vi "Dielectric vs Temperature - freq (4192A).vi"() -> ()   [LabVIEW 2013]
uses:
  <vilib>/Instr/_visa.llb/VISA Configure Serial Port (Instr).vi
  <vilib>/Utility/file.llb/Write To Spreadsheet File (DBL).vi
  Instance           5 32Saved   K vs Temp - freq (4284A) .vi
  Instance           6 32Saved   K vs Temp - freq (4284A) .vi
  Instance          15 32Saved   K vs Temp - freq (4284A) .vi
  Instance          16 32Saved   K vs Temp - freq (4284A) .vi
  Instance           7 32Saved   K vs Temp - freq (4284A) .vi
  Instance           8 32Saved   K vs Temp - freq (4284A) .vi
  Instance           9 32Saved   K vs Temp - freq (4284A) .vi
  Instance          10 32Saved   K vs Temp - freq (4284A) .vi
  Instance          11 32Saved   K vs Temp - freq (4284A) .vi
  Instance          12 32Saved   K vs Temp - freq (4284A) .vi
  Instance          13 32Saved   K vs Temp - freq (4284A) .vi
  Instance          14 32Saved   K vs Temp - freq (4284A) .vi
  Instance          17 32Saved   K vs Temp - freq (4284A) .vi
  Instance          18 32Saved   K vs Temp - freq (4284A) .vi
  Instance          19 32Saved   K vs Temp - freq (4284A) .vi
  Instance          20 32Saved   K vs Temp - freq (4284A) .vi
  Instance          21 32Saved   K vs Temp - freq (4284A) .vi
  Instance          22 32Saved   K vs Temp - freq (4284A) .vi
  Instance          23 32Saved   K vs Temp - freq (4284A) .vi
  Instance          25 32Saved   K vs Temp - freq (4284A) .vi
  Instance          24 32Saved   K vs Temp - freq (4284A) .vi
  Instance          26 32Saved   K vs Temp - freq (4284A) .vi
panel:
  in  "Freq Value (Hz) (1MHz)":dbl=1000000.0
  out "tand1M":dbl
  out "K1M":dbl
  out "C1M":dbl
  out "Temp1MHz":dbl format="%#_3g"
  in  "Freq Value (Hz) (500kHz)":dbl=500000.0
  out "tand500k":dbl
  out "K500k":dbl
  out "C500k":dbl
  out "Temp500kHz":dbl format="%#_3g"
  in  "Freq Value (Hz) (250kHz)":dbl=250000.0
  out "tand250k":dbl
  out "K250k":dbl
  out "C250k":dbl
  out "Temp250kHz":dbl format="%#_3g"
  in  "Freq Value (Hz) (100kHz)":dbl=100000.0
  out "tand100k":dbl
  out "K100k":dbl
  out "C100k":dbl
  out "Temp100kHz":dbl format="%#_3g"
  in  "Freq Value (Hz) (50kHz)":dbl=50000.0
  out "tand50k":dbl
  out "K50k":dbl
  out "C50k":dbl
  out "Temp50kHz":dbl format="%#_3g"
  in  "Freq Value (Hz) (25kHz)":dbl=25000.0
  out "tand25k":dbl
  out "K25k":dbl
  out "C25k":dbl
  out "Temp25kHz":dbl format="%#_3g"
  in  "Freq Value (Hz) (10kHz)":dbl=10000.0
  out "tand10k":dbl
  out "K10k":dbl
  out "C10k":dbl
  out "Temp10kHz":dbl format="%#_3g"
  in  "Freq Value (Hz) (5kHz)":dbl=5000.0
  out "tand5k":dbl
  out "K5k":dbl
  out "C5k":dbl
  out "Temp5kHz":dbl format="%#_3g"
  in  "Freq Value (Hz) (2.5kHz)":dbl=2500.0
  out "tand2.5k":dbl
  out "K2.5k":dbl
  out "C2.5k":dbl
  out "Temp2.5kHz":dbl format="%#_3g"
  in  "Freq Value (Hz) (1kHz)":dbl=1000.0
  out "tand1k":dbl
  out "K1k":dbl
  out "C1k":dbl
  out "Temp1kHz":dbl format="%#_3g"
  in  "tand500k":dbl[](array[numeric])
  in  "K500k":dbl[](array[numeric])
  in  "Temp500k":dbl[](array[numeric])
  out "Temp500Hz":dbl format="%#_3g"
  out "C500":dbl
  out "?":dbl
  out "tand500":dbl
  in  "Freq Value (Hz) (500Hz)":dbl=500.0
  in  "Freq Value (Hz) (250Hz)":dbl=250.0
  in  "Freq Value (Hz) (100Hz)":dbl=100.0
  in  "Freq Value (Hz) (50Hz)":dbl=50.0
  in  "Freq Value (Hz) (25Hz)":dbl=25.0
  in  "tand100k":dbl[](array[numeric])
  in  "tand10k":dbl[](array[numeric])
  in  "tand1k":dbl[](array[numeric])
  in  "tand100":dbl[](array[numeric])
  in  "K100k":dbl[](array[numeric])
  in  "K10k":dbl[](array[numeric])
  in  "K1k":dbl[](array[numeric])
  in  "K100":dbl[](array[numeric])
  in  "Temp100k":dbl[](array[numeric])
  in  "Temp10k":dbl[](array[numeric])
  in  "Temp1k":dbl[](array[numeric])
  in  "Temp100":dbl[](array[numeric])
  out "Temp250Hz":dbl format="%#_3g"
  out "Temp100Hz":dbl format="%#_3g"
  out "tand25":dbl
  out "Temp50Hz":dbl format="%#_3g"
  in  "Start":bool
  out "Thickness":dbl
  out "Area":dbl
  in  "stop":bool
  out "tand250":dbl
  out "tand100":dbl
  out "tand50":dbl
  out "K250":dbl
  out "K100":dbl
  out "K50":dbl
  out "K25":dbl
  out "C250":dbl
  out "C100":dbl
  out "C50":dbl
  out "C25":dbl
  out "Temp25Hz":dbl format="%#_3g"
  out "Dielectric Loss vs. Temperature":cluster{"Y":dbl[], "Y":dbl[]}[](graph)
  out "Relative Permittivity vs. Temperature":cluster{"Y":dbl[], "Y":dbl[]}[](graph)
  in  "Comment (Sample's Name, compositions, whatever you want,..)":string
  in  "Thickness (mm)":dbl
  in  "Diameter (mm)":dbl
  in  "Path & File Name (*.txt)":path
  # "Temperature (C)"
  # "Frequency (Hz)"
  # "Capacitance (F)"
  # "Relative Permittivity"
  # "Dielectric Loss"
  # "Sample Details"
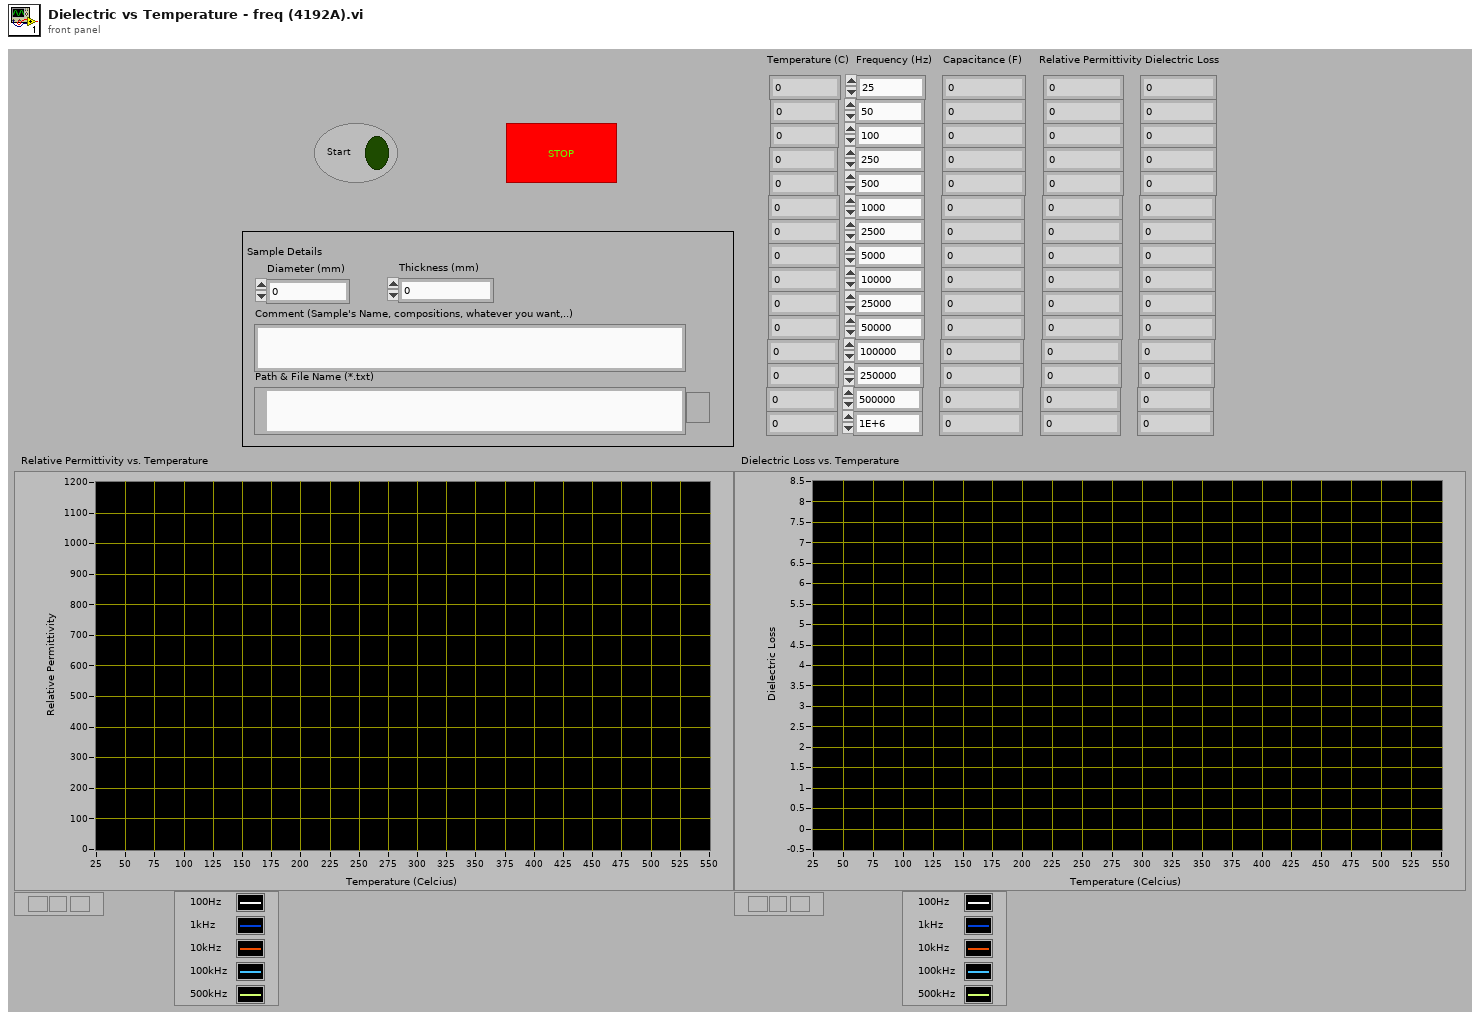
[diagram p1: front panel]
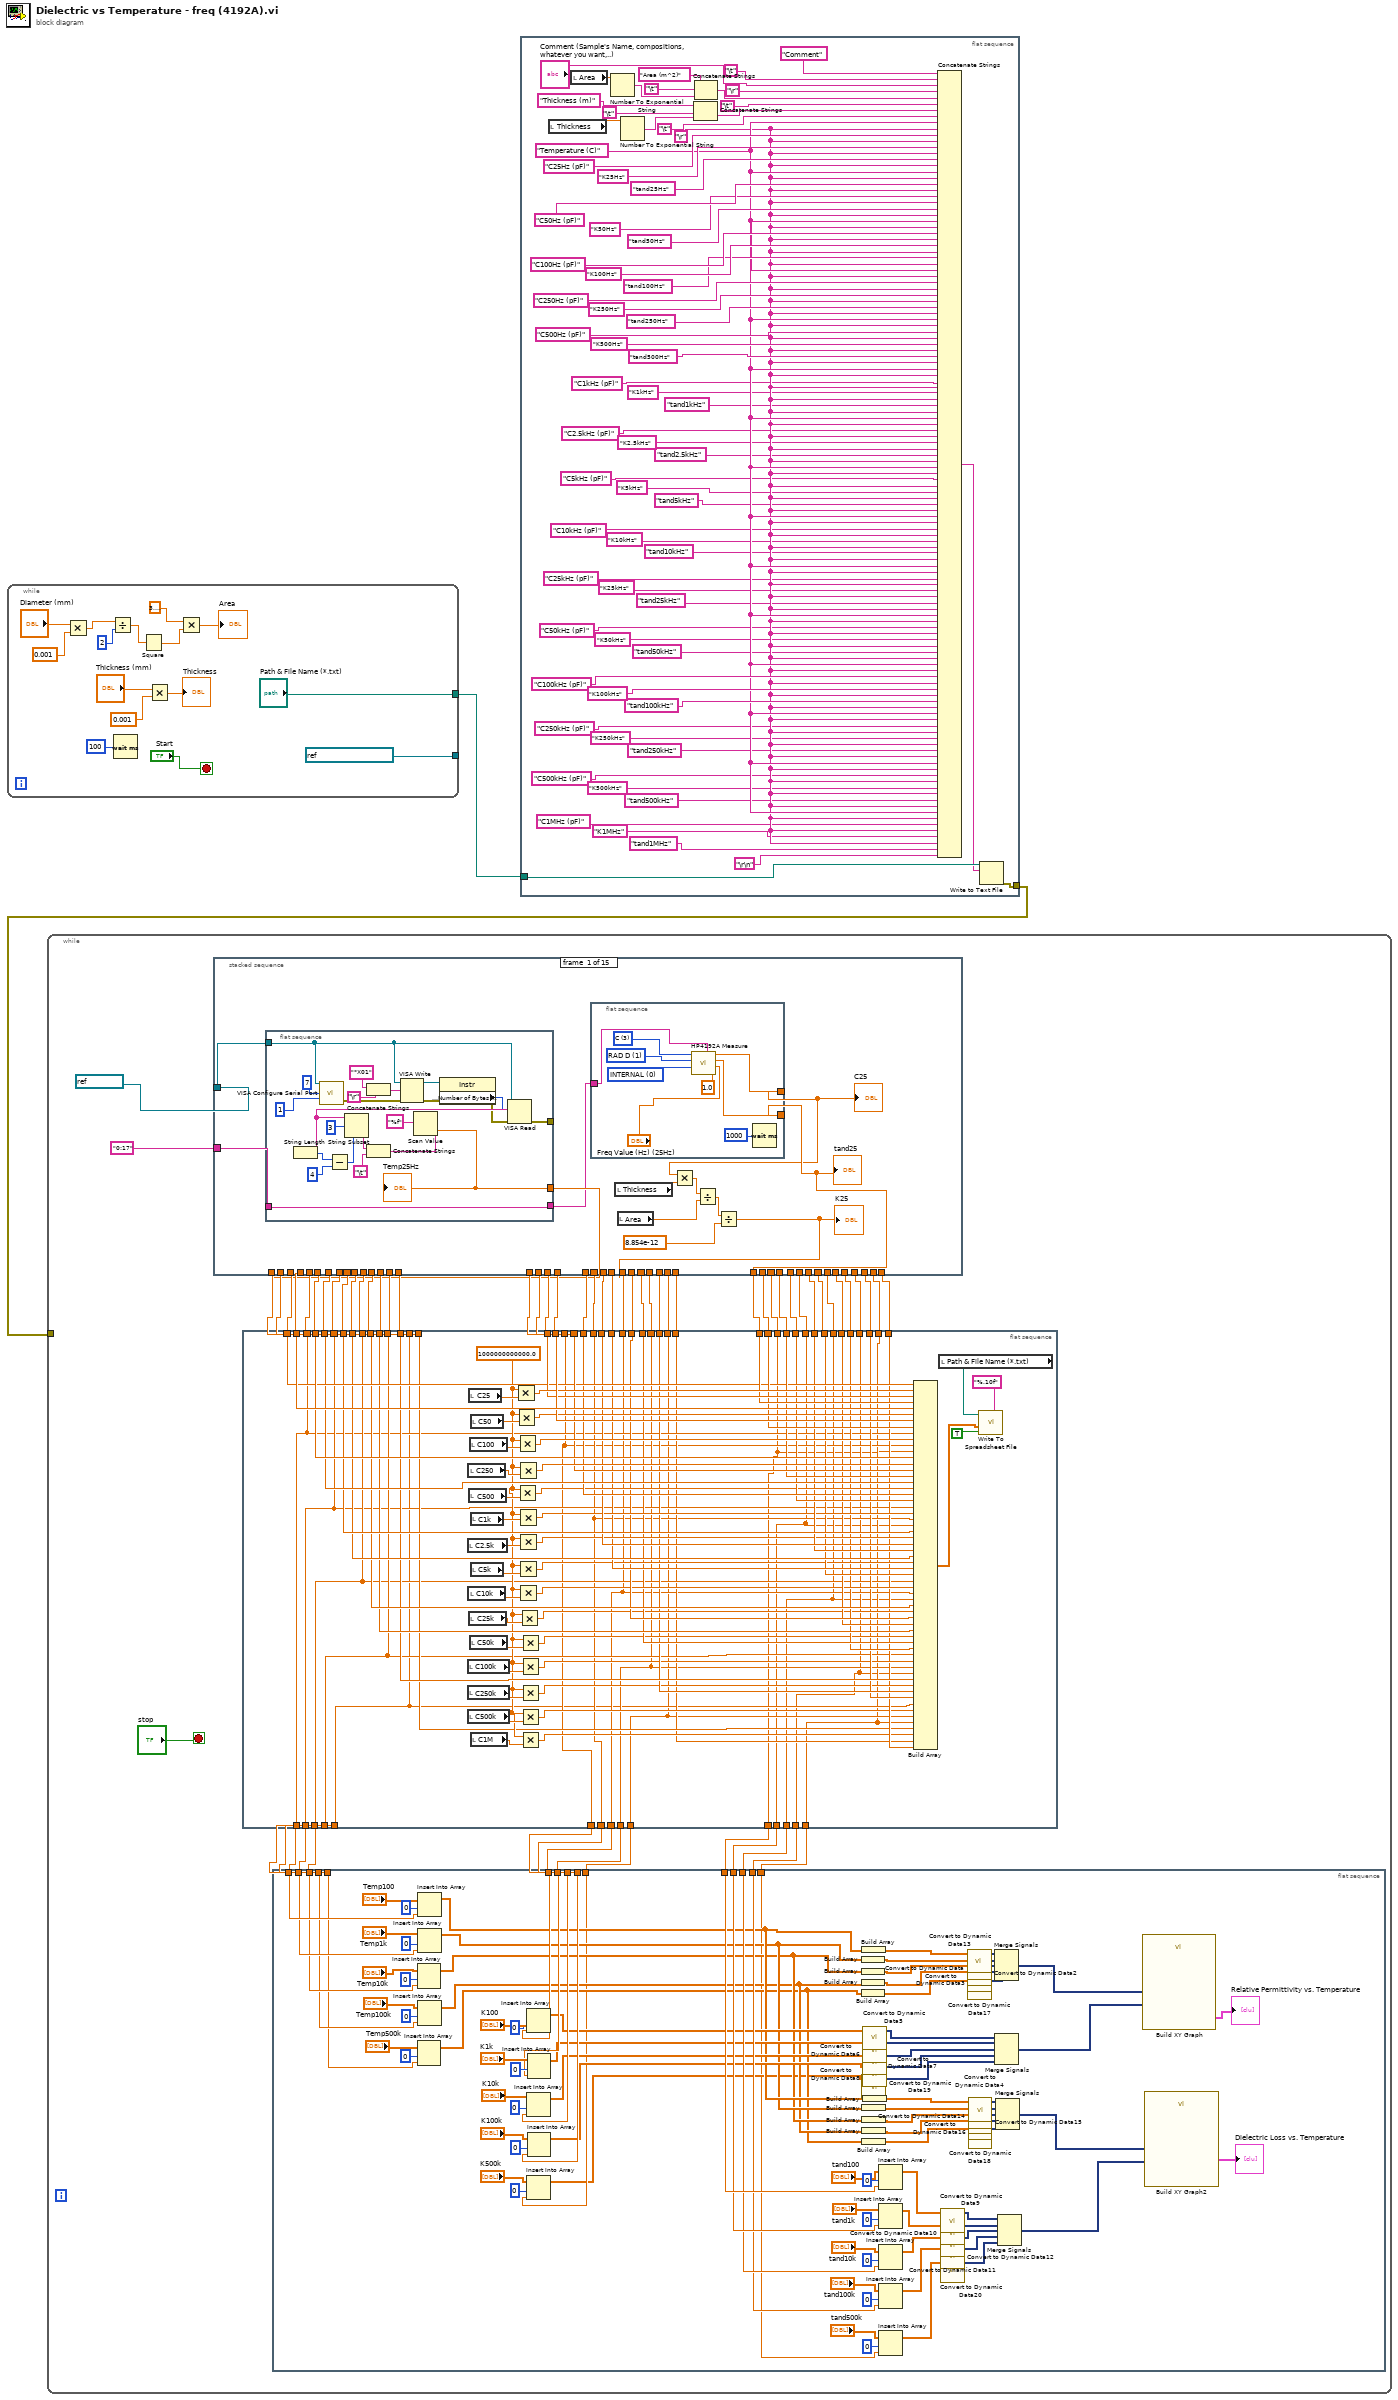
[diagram p0: block diagram]
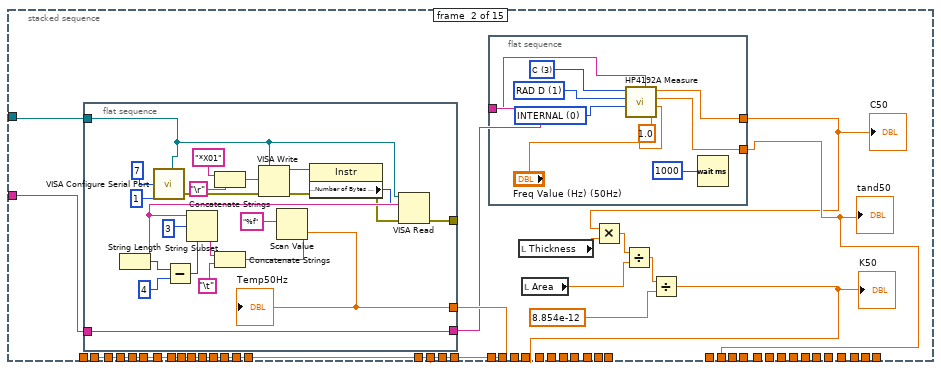
[diagram p2: hidden frame]
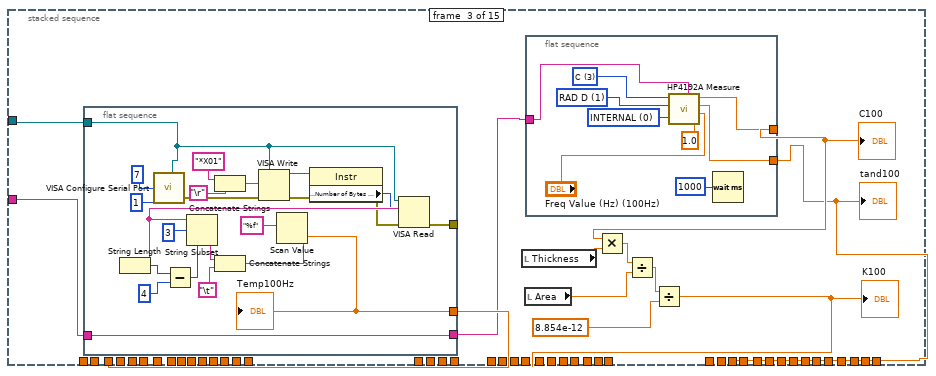
[diagram p3: hidden frame]
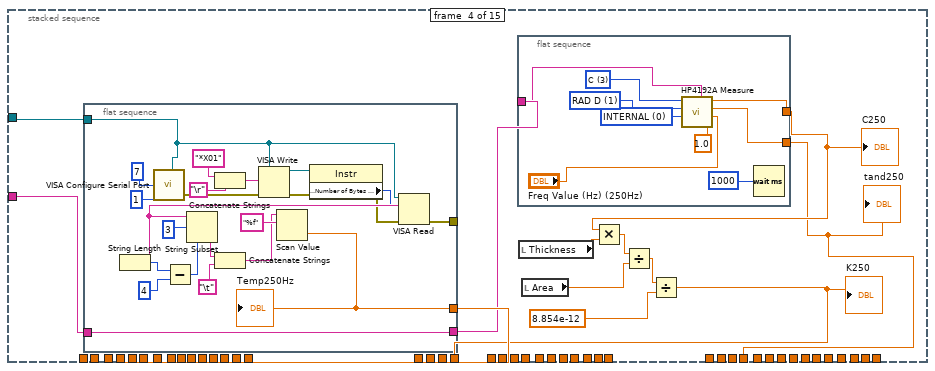
[diagram p4: hidden frame]
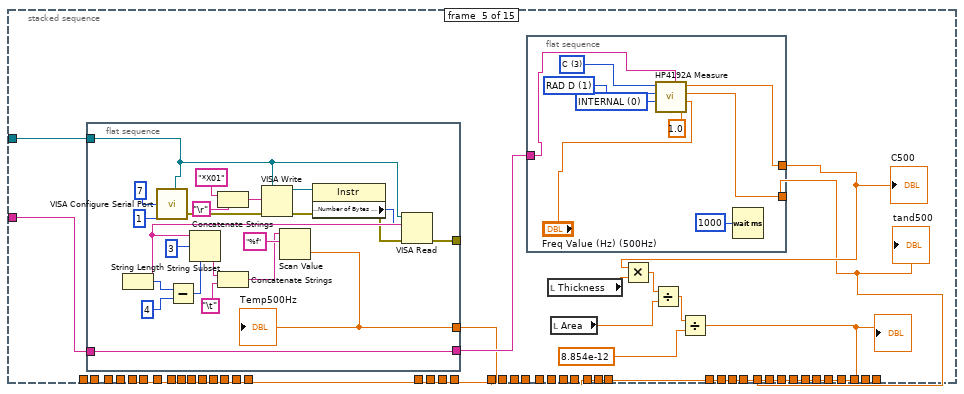
[diagram p5: hidden frame]
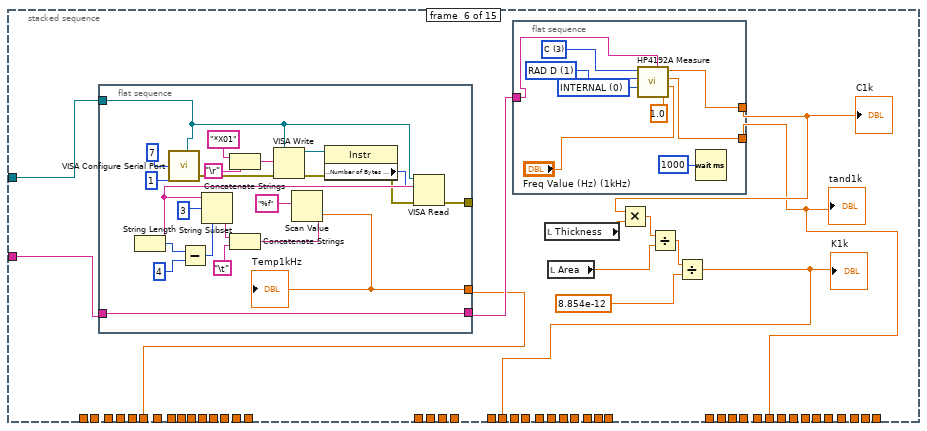
[diagram p6: hidden frame]
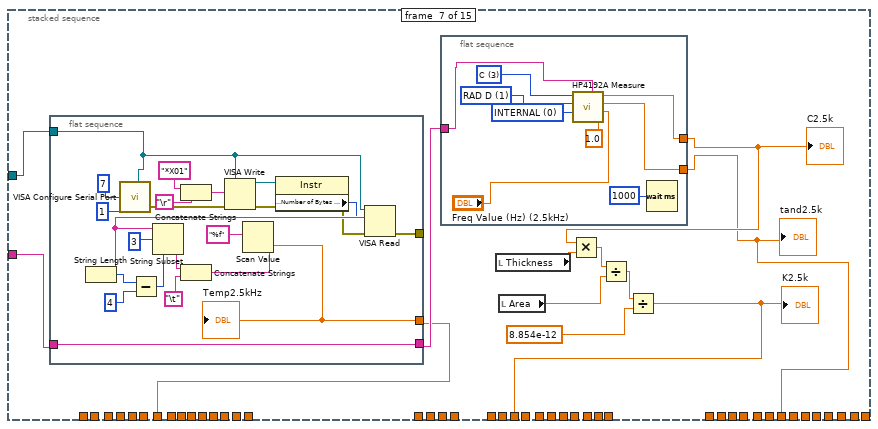
[diagram p7: hidden frame]
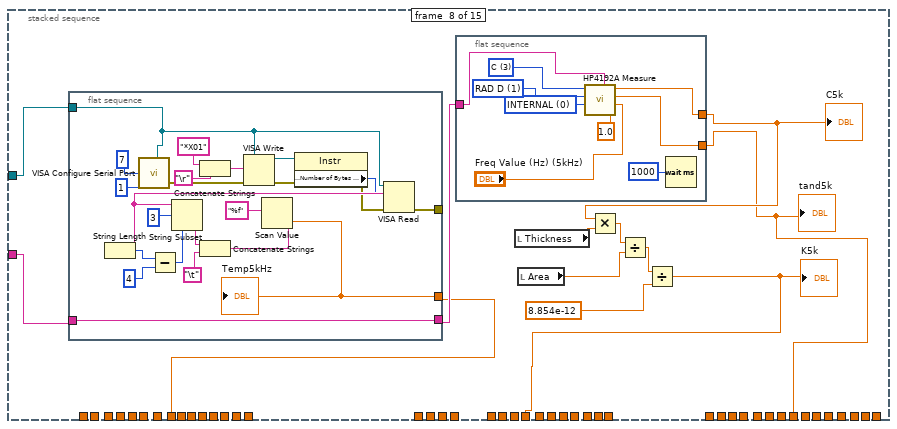
[diagram p8: hidden frame]
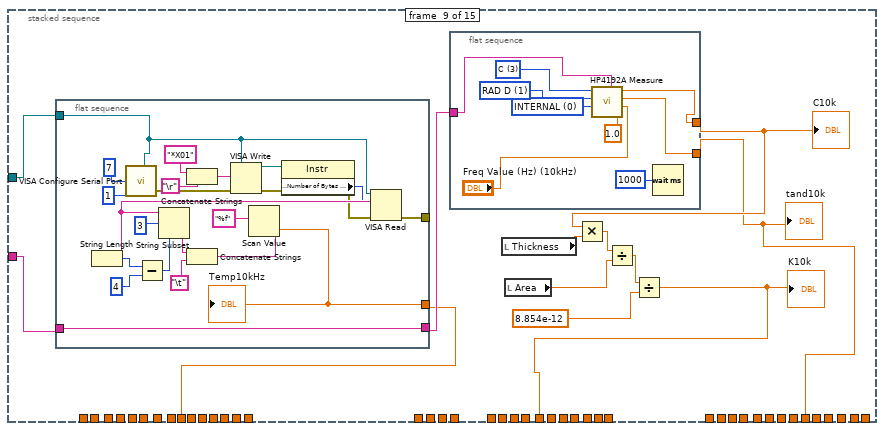
[diagram p9: hidden frame]
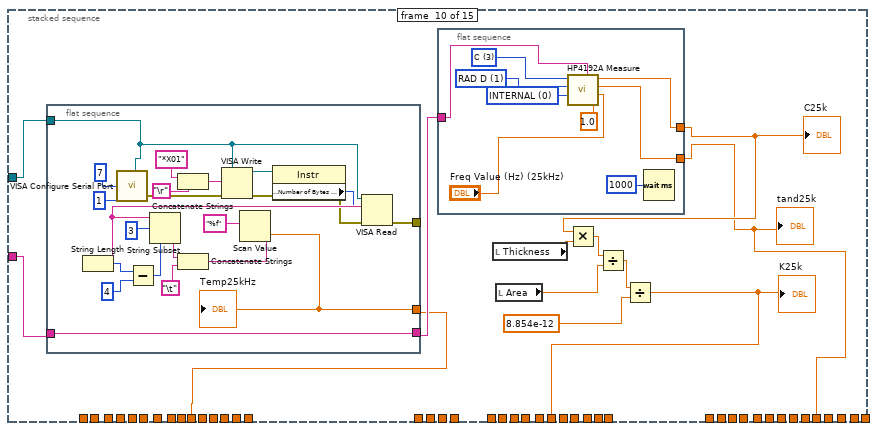
[diagram p10: hidden frame]
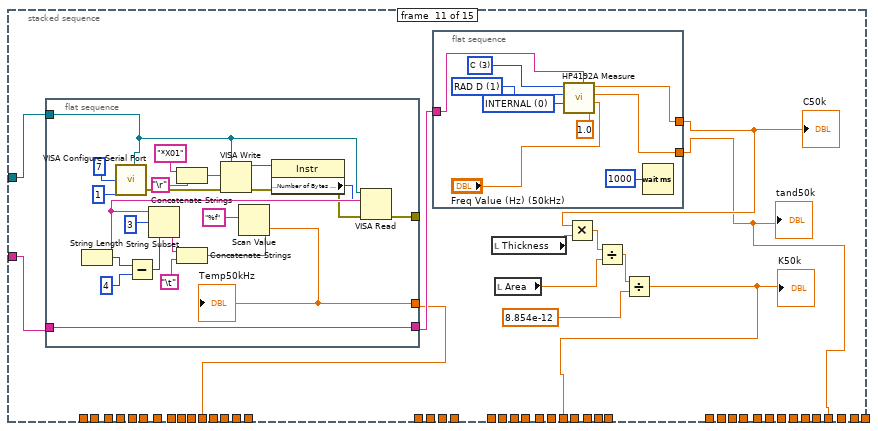
[diagram p11: hidden frame]
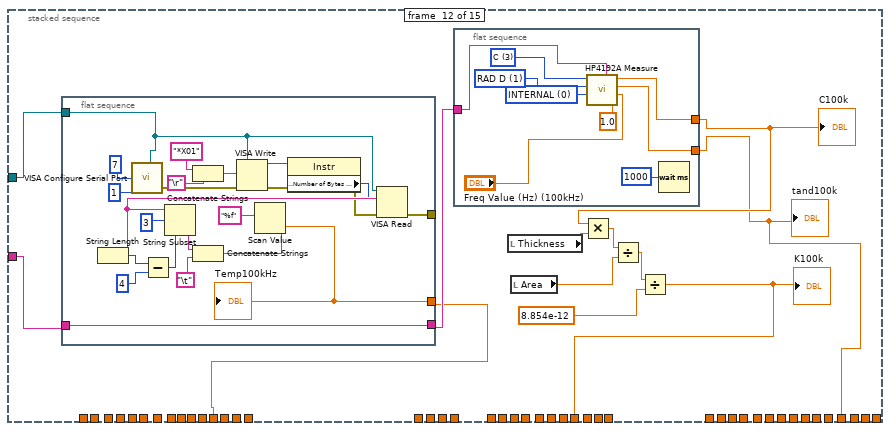
[diagram p12: hidden frame]
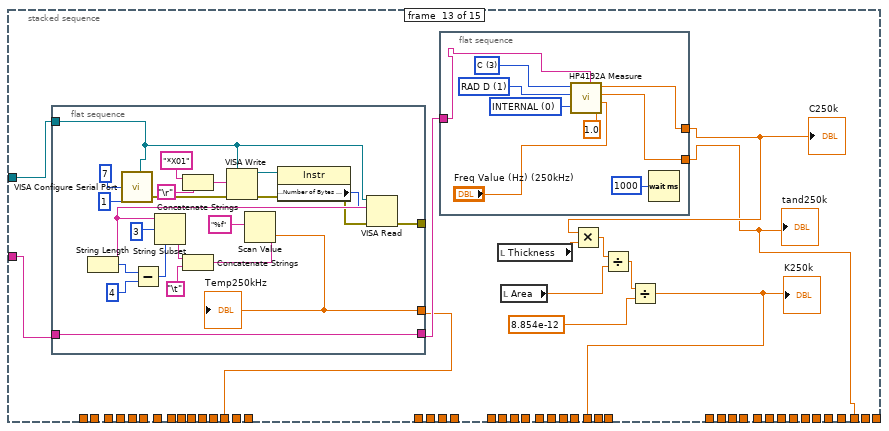
[diagram p13: hidden frame]
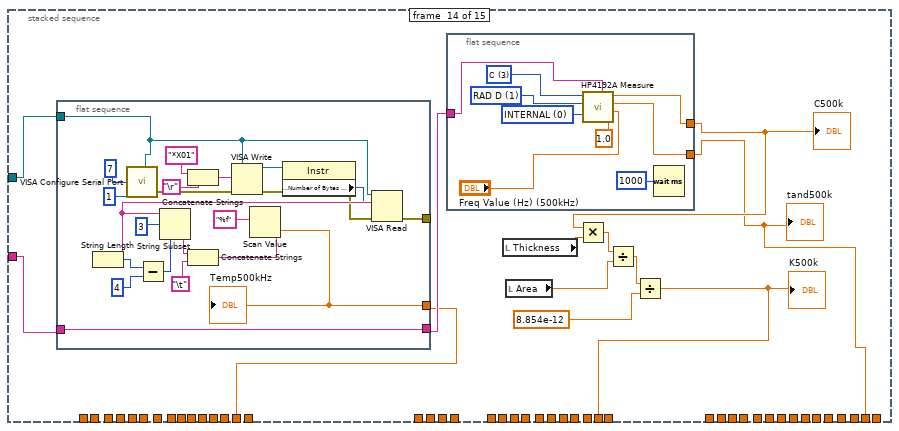
[diagram p14: hidden frame]
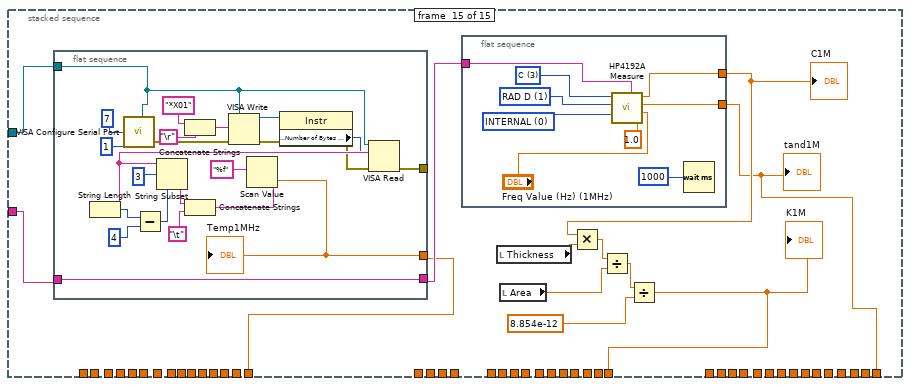
[diagram p15: hidden frame]
diagram:
  n1 = while {
    tunnel: ["Path & File Name (*.txt)"] -> w2
    tunnel: [refnum<visa-resource-name> "GPIB0::17::INSTR" ("VISA Omega (Serial - COM1)")] -> _
    stop <- "Start" stop-if-true
    n2 = Multiply(x="Diameter (mm)", y=0.001) -> (x*y=w12:dbl)
    n3 = Divide(x=w12, y=2) -> (x/y=w7:dbl)
    n4 = Wait (ms)(milliseconds to wait=u32 100) -> ()  [unwired: 1 out]
    n5 = Square(x=w7) -> (x^2=w8:dbl)
    n6 = Multiply(x="Thickness (mm)", y=0.001) -> (x*y=→"Thickness":dbl)
    n7 = Multiply(x=3.141592653589793, y=w8) -> (x*y=→"Area":dbl)
  }
  n8 = while {
    tunnel: w1 -> [_]
    stop <- "stop" stop-if-true
    n9 = stacked-sequence {
      tunnel: refnum<visa-resource-name> "COM1" ("VISA Omega (Serial - COM1)") -> [w268 w312 w356 w400 w437 w481 w525 w569 w613 w657 w701 w745 w789 w833 w877]
      tunnel: "0:17" -> [w267 w311 w355 w399 w438 w480 w524 w568 w612 w656 w700 w744 w788 w832 w876]
      tunnel: [w261 _ _ _ _ _ _ _ _ _ _ _ _ _ _] -> w68
      tunnel: [_ w305 _ _ _ _ _ _ _ _ _ _ _ _ _] -> w79
      tunnel: [_ _ w349 _ _ _ _ _ _ _ _ _ _ _ _] -> w78
      tunnel: [_ _ _ w393 _ _ _ _ _ _ _ _ _ _ _] -> w77
      tunnel: [w260 _ _ _ _ _ _ _ _ _ _ _ _ _ _] -> w76
      tunnel: [_ w304 _ _ _ _ _ _ _ _ _ _ _ _ _] -> w75
      tunnel: [_ _ w348 _ _ _ _ _ _ _ _ _ _ _ _] -> w74
      tunnel: [_ _ _ w392 _ _ _ _ _ _ _ _ _ _ _] -> w73
      tunnel: [w258 _ _ _ _ _ _ _ _ _ _ _ _ _ _] -> w72
      tunnel: [_ w303 _ _ _ _ _ _ _ _ _ _ _ _ _] -> w71
      tunnel: [_ _ w346 _ _ _ _ _ _ _ _ _ _ _ _] -> w70
      tunnel: [_ _ _ w389 _ _ _ _ _ _ _ _ _ _ _] -> w69
      tunnel: [_ _ _ _ w435 _ _ _ _ _ _ _ _ _ _] -> w67
      tunnel: [_ _ _ _ w434 _ _ _ _ _ _ _ _ _ _] -> w66
      tunnel: [_ _ _ _ w433 _ _ _ _ _ _ _ _ _ _] -> w65
      tunnel: [_ _ _ _ _ w479 _ _ _ _ _ _ _ _ _] -> w64
      tunnel: [_ _ _ _ _ w478 _ _ _ _ _ _ _ _ _] -> w63
      tunnel: [_ _ _ _ _ w477 _ _ _ _ _ _ _ _ _] -> w62
      tunnel: [_ _ _ _ _ _ w523 _ _ _ _ _ _ _ _] -> w61
      tunnel: [_ _ _ _ _ _ w522 _ _ _ _ _ _ _ _] -> w60
      tunnel: [_ _ _ _ _ _ w521 _ _ _ _ _ _ _ _] -> w59
      tunnel: [_ _ _ _ _ _ _ w567 _ _ _ _ _ _ _] -> w58
      tunnel: [_ _ _ _ _ _ _ w566 _ _ _ _ _ _ _] -> w57
      tunnel: [_ _ _ _ _ _ _ w565 _ _ _ _ _ _ _] -> w56
      tunnel: [_ _ _ _ _ _ _ _ w611 _ _ _ _ _ _] -> w55
      tunnel: [_ _ _ _ _ _ _ _ w610 _ _ _ _ _ _] -> w54
      tunnel: [_ _ _ _ _ _ _ _ w609 _ _ _ _ _ _] -> w53
      tunnel: [_ _ _ _ _ _ _ _ _ w655 _ _ _ _ _] -> w52
      tunnel: [_ _ _ _ _ _ _ _ _ w654 _ _ _ _ _] -> w51
      tunnel: [_ _ _ _ _ _ _ _ _ w653 _ _ _ _ _] -> w50
      tunnel: [_ _ _ _ _ _ _ _ _ _ w699 _ _ _ _] -> w49
      tunnel: [_ _ _ _ _ _ _ _ _ _ w698 _ _ _ _] -> w48
      tunnel: [_ _ _ _ _ _ _ _ _ _ w697 _ _ _ _] -> w47
      tunnel: [_ _ _ _ _ _ _ _ _ _ _ w743 _ _ _] -> w46
      tunnel: [_ _ _ _ _ _ _ _ _ _ _ w742 _ _ _] -> w45
      tunnel: [_ _ _ _ _ _ _ _ _ _ _ w741 _ _ _] -> w44
      tunnel: [_ _ _ _ _ _ _ _ _ _ _ _ w787 _ _] -> w43
      tunnel: [_ _ _ _ _ _ _ _ _ _ _ _ w786 _ _] -> w42
      tunnel: [_ _ _ _ _ _ _ _ _ _ _ _ w785 _ _] -> w41
      tunnel: [_ _ _ _ _ _ _ _ _ _ _ _ _ w831 _] -> w40
      tunnel: [_ _ _ _ _ _ _ _ _ _ _ _ _ w830 _] -> w39
      tunnel: [_ _ _ _ _ _ _ _ _ _ _ _ _ w829 _] -> w38
      tunnel: [_ _ _ _ _ _ _ _ _ _ _ _ _ _ w875] -> w35
      tunnel: [_ _ _ _ _ _ _ _ _ _ _ _ _ _ w874] -> w36
      tunnel: [_ _ _ _ _ _ _ _ _ _ _ _ _ _ w873] -> w37
      frame #0 {
        n10 = flat-sequence {
          tunnel: w268 -> [w281]
          tunnel: [w280] -> _
          tunnel: [w279] -> w261
          tunnel: w267 -> [w278]
          tunnel: [w278] -> w259
          frame #0 {
            n11 = call-poly "VISA Configure Serial Port"("VISA resource name"=w281, "data bits (8)"=7, "parity (0:none)"=1) -> ("error out"=w286:errorcluster)  [unwired: 11 in, 1 out]
            n12 = Concatenate Strings("*X01", "\r") -> (w289:string)
            n13 = VISA Write(VISA resource name=w281, write buffer=w289, error in (no error)=w286) -> (VISA resource name out=w300:refnum<visa-resource-name>, error out=w290:errorcluster)  [unwired: 1 out]
            n14 = property class="Instr"(reference=w300, error in=w290) -> (error out=w291:errorcluster, "Serial Settings:Number of Bytes at Serial Port"=w292:u32)  [unwired: 1 out]
            n15 = VISA Read(VISA resource name=w281, byte count=w292, error in (no error)=w291) -> (read buffer=w293:string, error out=w280:errorcluster)  [unwired: 2 out]
            n16 = String Length(string=w293) -> (length=w295:i32)
            n17 = Subtract(x=w295, y=4) -> (x-y=w297:i32)
            n18 = String Subset(string=w293, offset (0)=3, length (rest)=w297) -> (substring=w298:string)
            n19 = Concatenate Strings(w298, "\t") -> (w282:string)
            n20 = Scan Value(string=w282, format string="%f") -> (value=w279:dbl)  [unwired: 1 in, 1 out]
            "Temp25Hz" <- w279
          }
        }
        n21 = flat-sequence {
          tunnel: w259 -> [w274]
          tunnel: [w272] -> w258
          tunnel: [w273] -> w257
          frame #0 {
            w269 = i16 1 items=["DEG Q", "RAD D", "         R/G"] ("function B (deg q:0)")
            w270 = i16 3 items=["Z/Y", "R/G", "L", "C"] ("function A (z/y:0)")
            w271 = i16 0 items=["INTERNAL", "EXTERNAL", "HOLD/MANUAL"] ("trigger (internal:0)")
            n22 = call "HP4192A Measure.vi"("OSC level (V)"=1.0, "test signal\nfreq (Hz)"="Freq Value (Hz) (25Hz)", "GPIB addess"=w274, "trigger (internal:0)"=w271, "function B (deg q:0)"=w269, "function A (z/y:0)"=w270) -> ("display B"=w272:dbl, "display A"=w273:dbl)  [unwired: 4 in]
            n23 = Wait (ms)(milliseconds to wait=u32 1000) -> ()  [unwired: 1 out]
          }
        }
        n24 = local read "Thickness"() -> (w266:dbl)
        n25 = local read "Area"() -> (w264:dbl)
        n26 = Multiply(x=w257, y=w266) -> (x*y=w265:dbl)
        n27 = Divide(x=w265, y=w264) -> (x/y=w263:dbl)
        n28 = Divide(x=w263, y=8.854e-12) -> (x/y=w260:dbl)
        "K25" <- w260
        "C25" <- w257
        "tand25" <- w258
      }
      frame #1 {
        n29 = flat-sequence {
          tunnel: w312 -> [w325]
          tunnel: [w324] -> _
          tunnel: [w323] -> w305
          tunnel: w311 -> [w322]
          tunnel: [w322] -> w301
          frame #0 {
            n30 = call-poly "VISA Configure Serial Port"("VISA resource name"=w325, "data bits (8)"=7, "parity (0:none)"=1) -> ("error out"=w330:errorcluster)  [unwired: 11 in, 1 out]
            n31 = Concatenate Strings("*X01", "\r") -> (w333:string)
            n32 = VISA Write(VISA resource name=w325, write buffer=w333, error in (no error)=w330) -> (VISA resource name out=w344:refnum<visa-resource-name>, error out=w334:errorcluster)  [unwired: 1 out]
            n33 = property class="Instr"(reference=w344, error in=w334) -> (error out=w335:errorcluster, "Serial Settings:Number of Bytes at Serial Port"=w336:u32)  [unwired: 1 out]
            n34 = VISA Read(VISA resource name=w325, byte count=w336, error in (no error)=w335) -> (read buffer=w337:string, error out=w324:errorcluster)  [unwired: 2 out]
            n35 = String Length(string=w337) -> (length=w339:i32)
            n36 = Subtract(x=w339, y=4) -> (x-y=w341:i32)
            n37 = String Subset(string=w337, offset (0)=3, length (rest)=w341) -> (substring=w342:string)
            n38 = Concatenate Strings(w342, "\t") -> (w326:string)
            n39 = Scan Value(string=w326, format string="%f") -> (value=w323:dbl)  [unwired: 1 in, 1 out]
            "Temp50Hz" <- w323
          }
        }
        n40 = flat-sequence {
          tunnel: w301 -> [w316]
          tunnel: [w314] -> w303
          tunnel: [w315] -> w302
          frame #0 {
            w313 = i16 0 items=["INTERNAL", "EXTERNAL", "HOLD/MANUAL"] ("trigger (internal:0)")
            w319 = i16 1 items=["DEG Q", "RAD D", "         R/G"] ("function B (deg q:0)")
            w320 = i16 3 items=["Z/Y", "R/G", "L", "C"] ("function A (z/y:0)")
            n41 = call "HP4192A Measure.vi"("OSC level (V)"=1.0, "test signal\nfreq (Hz)"="Freq Value (Hz) (50Hz)", "GPIB addess"=w316, "trigger (internal:0)"=w313, "function B (deg q:0)"=w319, "function A (z/y:0)"=w320) -> ("display B"=w314:dbl, "display A"=w315:dbl)  [unwired: 4 in]
            n42 = Wait (ms)(milliseconds to wait=u32 1000) -> ()  [unwired: 1 out]
          }
        }
        n43 = local read "Thickness"() -> (w310:dbl)
        n44 = local read "Area"() -> (w308:dbl)
        n45 = Multiply(x=w302, y=w310) -> (x*y=w309:dbl)
        n46 = Divide(x=w309, y=w308) -> (x/y=w307:dbl)
        n47 = Divide(x=w307, y=8.854e-12) -> (x/y=w304:dbl)
        "K50" <- w304
        "tand50" <- w303
        "C50" <- w302
      }
      frame #2 {
        n48 = flat-sequence {
          tunnel: w356 -> [w369]
          tunnel: [w368] -> _
          tunnel: [w367] -> w349
          tunnel: w355 -> [w366]
          tunnel: [w366] -> w345
          frame #0 {
            n49 = call-poly "VISA Configure Serial Port"("VISA resource name"=w369, "data bits (8)"=7, "parity (0:none)"=1) -> ("error out"=w374:errorcluster)  [unwired: 11 in, 1 out]
            n50 = Concatenate Strings("*X01", "\r") -> (w377:string)
            n51 = VISA Write(VISA resource name=w369, write buffer=w377, error in (no error)=w374) -> (VISA resource name out=w388:refnum<visa-resource-name>, error out=w378:errorcluster)  [unwired: 1 out]
            n52 = property class="Instr"(reference=w388, error in=w378) -> (error out=w379:errorcluster, "Serial Settings:Number of Bytes at Serial Port"=w380:u32)  [unwired: 1 out]
            n53 = VISA Read(VISA resource name=w369, byte count=w380, error in (no error)=w379) -> (read buffer=w381:string, error out=w368:errorcluster)  [unwired: 2 out]
            n54 = String Length(string=w381) -> (length=w383:i32)
            n55 = Subtract(x=w383, y=4) -> (x-y=w385:i32)
            n56 = String Subset(string=w381, offset (0)=3, length (rest)=w385) -> (substring=w386:string)
            n57 = Concatenate Strings(w386, "\t") -> (w370:string)
            n58 = Scan Value(string=w370, format string="%f") -> (value=w367:dbl)  [unwired: 1 in, 1 out]
            "Temp100Hz" <- w367
          }
        }
        n59 = local read "Thickness"() -> (w354:dbl)
        n60 = local read "Area"() -> (w352:dbl)
        n61 = flat-sequence {
          tunnel: w345 -> [w360]
          tunnel: [w358] -> w346
          tunnel: [w359] -> w347
          frame #0 {
            w357 = i16 0 items=["INTERNAL", "EXTERNAL", "HOLD/MANUAL"] ("trigger (internal:0)")
            w363 = i16 1 items=["DEG Q", "RAD D", "         R/G"] ("function B (deg q:0)")
            w364 = i16 3 items=["Z/Y", "R/G", "L", "C"] ("function A (z/y:0)")
            n62 = call "HP4192A Measure.vi"("OSC level (V)"=1.0, "test signal\nfreq (Hz)"="Freq Value (Hz) (100Hz)", "GPIB addess"=w360, "trigger (internal:0)"=w357, "function B (deg q:0)"=w363, "function A (z/y:0)"=w364) -> ("display B"=w358:dbl, "display A"=w359:dbl)  [unwired: 4 in]
            n63 = Wait (ms)(milliseconds to wait=u32 1000) -> ()  [unwired: 1 out]
          }
        }
        n64 = Multiply(x=w347, y=w354) -> (x*y=w353:dbl)
        n65 = Divide(x=w353, y=w352) -> (x/y=w351:dbl)
        n66 = Divide(x=w351, y=8.854e-12) -> (x/y=w348:dbl)
        "K100" <- w348
        "C100" <- w347
        "tand100" <- w346
      }
      frame #3 {
        n67 = flat-sequence {
          tunnel: w400 -> [w413]
          tunnel: [w412] -> _
          tunnel: [w411] -> w393
          tunnel: w399 -> [w410]
          tunnel: [w410] -> w391
          frame #0 {
            n68 = call-poly "VISA Configure Serial Port"("VISA resource name"=w413, "data bits (8)"=7, "parity (0:none)"=1) -> ("error out"=w418:errorcluster)  [unwired: 11 in, 1 out]
            n69 = Concatenate Strings("*X01", "\r") -> (w421:string)
            n70 = VISA Write(VISA resource name=w413, write buffer=w421, error in (no error)=w418) -> (VISA resource name out=w432:refnum<visa-resource-name>, error out=w422:errorcluster)  [unwired: 1 out]
            n71 = property class="Instr"(reference=w432, error in=w422) -> (error out=w423:errorcluster, "Serial Settings:Number of Bytes at Serial Port"=w424:u32)  [unwired: 1 out]
            n72 = VISA Read(VISA resource name=w413, byte count=w424, error in (no error)=w423) -> (read buffer=w425:string, error out=w412:errorcluster)  [unwired: 2 out]
            n73 = String Length(string=w425) -> (length=w427:i32)
            n74 = Subtract(x=w427, y=4) -> (x-y=w429:i32)
            n75 = String Subset(string=w425, offset (0)=3, length (rest)=w429) -> (substring=w430:string)
            n76 = Concatenate Strings(w430, "\t") -> (w414:string)
            n77 = Scan Value(string=w414, format string="%f") -> (value=w411:dbl)  [unwired: 1 in, 1 out]
            "Temp250Hz" <- w411
          }
        }
        n78 = flat-sequence {
          tunnel: w391 -> [w404]
          tunnel: [w402] -> w389
          tunnel: [w403] -> w390
          frame #0 {
            w401 = i16 0 items=["INTERNAL", "EXTERNAL", "HOLD/MANUAL"] ("trigger (internal:0)")
            w407 = i16 1 items=["DEG Q", "RAD D", "         R/G"] ("function B (deg q:0)")
            w408 = i16 3 items=["Z/Y", "R/G", "L", "C"] ("function A (z/y:0)")
            n79 = call "HP4192A Measure.vi"("OSC level (V)"=1.0, "test signal\nfreq (Hz)"="Freq Value (Hz) (250Hz)", "GPIB addess"=w404, "trigger (internal:0)"=w401, "function B (deg q:0)"=w407, "function A (z/y:0)"=w408) -> ("display B"=w402:dbl, "display A"=w403:dbl)  [unwired: 4 in]
            n80 = Wait (ms)(milliseconds to wait=u32 1000) -> ()  [unwired: 1 out]
          }
        }
        n81 = local read "Thickness"() -> (w398:dbl)
        n82 = local read "Area"() -> (w396:dbl)
        n83 = Multiply(x=w390, y=w398) -> (x*y=w397:dbl)
        n84 = Divide(x=w397, y=w396) -> (x/y=w395:dbl)
        n85 = Divide(x=w395, y=8.854e-12) -> (x/y=w392:dbl)
        "K250" <- w392
        "C250" <- w390
        "tand250" <- w389
      }
      frame #4 {
        n86 = flat-sequence {
          tunnel: w437 -> [w457]
          tunnel: [w456] -> _
          tunnel: [w455] -> w435
          tunnel: w438 -> [w454]
          tunnel: [w454] -> w436
          frame #0 {
            n87 = call-poly "VISA Configure Serial Port"("VISA resource name"=w457, "data bits (8)"=7, "parity (0:none)"=1) -> ("error out"=w462:errorcluster)  [unwired: 11 in, 1 out]
            n88 = Concatenate Strings("*X01", "\r") -> (w465:string)
            n89 = VISA Write(VISA resource name=w457, write buffer=w465, error in (no error)=w462) -> (VISA resource name out=w476:refnum<visa-resource-name>, error out=w466:errorcluster)  [unwired: 1 out]
            n90 = property class="Instr"(reference=w476, error in=w466) -> (error out=w467:errorcluster, "Serial Settings:Number of Bytes at Serial Port"=w468:u32)  [unwired: 1 out]
            n91 = VISA Read(VISA resource name=w457, byte count=w468, error in (no error)=w467) -> (read buffer=w469:string, error out=w456:errorcluster)  [unwired: 2 out]
            n92 = String Length(string=w469) -> (length=w471:i32)
            n93 = Subtract(x=w471, y=4) -> (x-y=w473:i32)
            n94 = String Subset(string=w469, offset (0)=3, length (rest)=w473) -> (substring=w474:string)
            n95 = Concatenate Strings(w474, "\t") -> (w458:string)
            n96 = Scan Value(string=w458, format string="%f") -> (value=w455:dbl)  [unwired: 1 in, 1 out]
            "Temp500Hz" <- w455
          }
        }
        n97 = flat-sequence {
          tunnel: w436 -> [w446]
          tunnel: [w448] -> w433
          tunnel: [w447] -> w439
          frame #0 {
            w445 = i16 0 items=["INTERNAL", "EXTERNAL", "HOLD/MANUAL"] ("trigger (internal:0)")
            w451 = i16 1 items=["DEG Q", "RAD D", "         R/G"] ("function B (deg q:0)")
            w452 = i16 3 items=["Z/Y", "R/G", "L", "C"] ("function A (z/y:0)")
            n98 = call "HP4192A Measure.vi"("OSC level (V)"=1.0, "test signal\nfreq (Hz)"="Freq Value (Hz) (500Hz)", "GPIB addess"=w446, "trigger (internal:0)"=w445, "function B (deg q:0)"=w451, "function A (z/y:0)"=w452) -> ("display B"=w448:dbl, "display A"=w447:dbl)  [unwired: 4 in]
            n99 = Wait (ms)(milliseconds to wait=u32 1000) -> ()  [unwired: 1 out]
          }
        }
        n100 = local read "Thickness"() -> (w444:dbl)
        n101 = local read "Area"() -> (w442:dbl)
        n102 = Multiply(x=w439, y=w444) -> (x*y=w443:dbl)
        n103 = Divide(x=w443, y=w442) -> (x/y=w441:dbl)
        n104 = Divide(x=w441, y=8.854e-12) -> (x/y=w434:dbl)
        "?" <- w434
        "C500" <- w439
        "tand500" <- w433
      }
      frame #5 {
        n105 = flat-sequence {
          tunnel: w481 -> [w501]
          tunnel: [w500] -> _
          tunnel: [w499] -> w479
          tunnel: w480 -> [w498]
          tunnel: [w498] -> w483
          frame #0 {
            n106 = call-poly "VISA Configure Serial Port"("VISA resource name"=w501, "data bits (8)"=7, "parity (0:none)"=1) -> ("error out"=w506:errorcluster)  [unwired: 11 in, 1 out]
            n107 = Concatenate Strings("*X01", "\r") -> (w509:string)
            n108 = VISA Write(VISA resource name=w501, write buffer=w509, error in (no error)=w506) -> (VISA resource name out=w520:refnum<visa-resource-name>, error out=w510:errorcluster)  [unwired: 1 out]
            n109 = property class="Instr"(reference=w520, error in=w510) -> (error out=w511:errorcluster, "Serial Settings:Number of Bytes at Serial Port"=w512:u32)  [unwired: 1 out]
            n110 = VISA Read(VISA resource name=w501, byte count=w512, error in (no error)=w511) -> (read buffer=w513:string, error out=w500:errorcluster)  [unwired: 2 out]
            n111 = String Length(string=w513) -> (length=w515:i32)
            n112 = Subtract(x=w515, y=4) -> (x-y=w517:i32)
            n113 = String Subset(string=w513, offset (0)=3, length (rest)=w517) -> (substring=w518:string)
            n114 = Concatenate Strings(w518, "\t") -> (w502:string)
            n115 = Scan Value(string=w502, format string="%f") -> (value=w499:dbl)  [unwired: 1 in, 1 out]
            "Temp1kHz" <- w499
          }
        }
        n116 = flat-sequence {
          tunnel: w483 -> [w493]
          tunnel: [w490] -> w477
          tunnel: [w491] -> w482
          frame #0 {
            w489 = i16 0 items=["INTERNAL", "EXTERNAL", "HOLD/MANUAL"] ("trigger (internal:0)")
            w495 = i16 1 items=["DEG Q", "RAD D", "         R/G"] ("function B (deg q:0)")
            w496 = i16 3 items=["Z/Y", "R/G", "L", "C"] ("function A (z/y:0)")
            n117 = call "HP4192A Measure.vi"("OSC level (V)"=1.0, "test signal\nfreq (Hz)"="Freq Value (Hz) (1kHz)", "GPIB addess"=w493, "trigger (internal:0)"=w489, "function B (deg q:0)"=w495, "function A (z/y:0)"=w496) -> ("display B"=w490:dbl, "display A"=w491:dbl)  [unwired: 4 in]
            n118 = Wait (ms)(milliseconds to wait=u32 1000) -> ()  [unwired: 1 out]
          }
        }
        n119 = local read "Thickness"() -> (w488:dbl)
        n120 = local read "Area"() -> (w486:dbl)
        n121 = Multiply(x=w482, y=w488) -> (x*y=w487:dbl)
        n122 = Divide(x=w487, y=w486) -> (x/y=w485:dbl)
        n123 = Divide(x=w485, y=8.854e-12) -> (x/y=w478:dbl)
        "K1k" <- w478
        "C1k" <- w482
        "tand1k" <- w477
      }
      frame #6 {
        n124 = flat-sequence {
          tunnel: w525 -> [w545]
          tunnel: [w544] -> _
          tunnel: [w543] -> w523
          tunnel: w524 -> [w542]
          tunnel: [w542] -> w527
          frame #0 {
            n125 = call-poly "VISA Configure Serial Port"("VISA resource name"=w545, "data bits (8)"=7, "parity (0:none)"=1) -> ("error out"=w550:errorcluster)  [unwired: 11 in, 1 out]
            n126 = Concatenate Strings("*X01", "\r") -> (w553:string)
            n127 = VISA Write(VISA resource name=w545, write buffer=w553, error in (no error)=w550) -> (VISA resource name out=w564:refnum<visa-resource-name>, error out=w554:errorcluster)  [unwired: 1 out]
            n128 = property class="Instr"(reference=w564, error in=w554) -> (error out=w555:errorcluster, "Serial Settings:Number of Bytes at Serial Port"=w556:u32)  [unwired: 1 out]
            n129 = VISA Read(VISA resource name=w545, byte count=w556, error in (no error)=w555) -> (read buffer=w557:string, error out=w544:errorcluster)  [unwired: 2 out]
            n130 = String Length(string=w557) -> (length=w559:i32)
            n131 = Subtract(x=w559, y=4) -> (x-y=w561:i32)
            n132 = String Subset(string=w557, offset (0)=3, length (rest)=w561) -> (substring=w562:string)
            n133 = Concatenate Strings(w562, "\t") -> (w546:string)
            n134 = Scan Value(string=w546, format string="%f") -> (value=w543:dbl)  [unwired: 1 in, 1 out]
            "Temp2.5kHz" <- w543
          }
        }
        n135 = flat-sequence {
          tunnel: w527 -> [w534]
          tunnel: [w536] -> w521
          tunnel: [w535] -> w526
          frame #0 {
            w533 = i16 0 items=["INTERNAL", "EXTERNAL", "HOLD/MANUAL"] ("trigger (internal:0)")
            w539 = i16 1 items=["DEG Q", "RAD D", "         R/G"] ("function B (deg q:0)")
            w540 = i16 3 items=["Z/Y", "R/G", "L", "C"] ("function A (z/y:0)")
            n136 = call "HP4192A Measure.vi"("OSC level (V)"=1.0, "test signal\nfreq (Hz)"="Freq Value (Hz) (2.5kHz)", "GPIB addess"=w534, "trigger (internal:0)"=w533, "function B (deg q:0)"=w539, "function A (z/y:0)"=w540) -> ("display B"=w536:dbl, "display A"=w535:dbl)  [unwired: 4 in]
            n137 = Wait (ms)(milliseconds to wait=u32 1000) -> ()  [unwired: 1 out]
          }
        }
        n138 = local read "Thickness"() -> (w532:dbl)
        n139 = local read "Area"() -> (w530:dbl)
        n140 = Multiply(x=w526, y=w532) -> (x*y=w531:dbl)
        n141 = Divide(x=w531, y=w530) -> (x/y=w529:dbl)
        n142 = Divide(x=w529, y=8.854e-12) -> (x/y=w522:dbl)
        "K2.5k" <- w522
        "C2.5k" <- w526
        "tand2.5k" <- w521
      }
      frame #7 {
        n143 = flat-sequence {
          tunnel: w569 -> [w589]
          tunnel: [w588] -> _
          tunnel: [w587] -> w567
          tunnel: w568 -> [w586]
          tunnel: [w586] -> w571
          frame #0 {
            n144 = call-poly "VISA Configure Serial Port"("VISA resource name"=w589, "data bits (8)"=7, "parity (0:none)"=1) -> ("error out"=w594:errorcluster)  [unwired: 11 in, 1 out]
            n145 = Concatenate Strings("*X01", "\r") -> (w597:string)
            n146 = VISA Write(VISA resource name=w589, write buffer=w597, error in (no error)=w594) -> (VISA resource name out=w608:refnum<visa-resource-name>, error out=w598:errorcluster)  [unwired: 1 out]
            n147 = property class="Instr"(reference=w608, error in=w598) -> (error out=w599:errorcluster, "Serial Settings:Number of Bytes at Serial Port"=w600:u32)  [unwired: 1 out]
            n148 = VISA Read(VISA resource name=w589, byte count=w600, error in (no error)=w599) -> (read buffer=w601:string, error out=w588:errorcluster)  [unwired: 2 out]
            n149 = String Length(string=w601) -> (length=w603:i32)
            n150 = Subtract(x=w603, y=4) -> (x-y=w605:i32)
            n151 = String Subset(string=w601, offset (0)=3, length (rest)=w605) -> (substring=w606:string)
            n152 = Concatenate Strings(w606, "\t") -> (w590:string)
            n153 = Scan Value(string=w590, format string="%f") -> (value=w587:dbl)  [unwired: 1 in, 1 out]
            "Temp5kHz" <- w587
          }
        }
        n154 = flat-sequence {
          tunnel: w571 -> [w578]
          tunnel: [w580] -> w565
          tunnel: [w579] -> w570
          frame #0 {
            w577 = i16 0 items=["INTERNAL", "EXTERNAL", "HOLD/MANUAL"] ("trigger (internal:0)")
            w583 = i16 1 items=["DEG Q", "RAD D", "         R/G"] ("function B (deg q:0)")
            w584 = i16 3 items=["Z/Y", "R/G", "L", "C"] ("function A (z/y:0)")
            n155 = call "HP4192A Measure.vi"("OSC level (V)"=1.0, "test signal\nfreq (Hz)"="Freq Value (Hz) (5kHz)", "GPIB addess"=w578, "trigger (internal:0)"=w577, "function B (deg q:0)"=w583, "function A (z/y:0)"=w584) -> ("display B"=w580:dbl, "display A"=w579:dbl)  [unwired: 4 in]
            n156 = Wait (ms)(milliseconds to wait=u32 1000) -> ()  [unwired: 1 out]
          }
        }
        n157 = local read "Thickness"() -> (w576:dbl)
        n158 = local read "Area"() -> (w574:dbl)
        n159 = Multiply(x=w570, y=w576) -> (x*y=w575:dbl)
        n160 = Divide(x=w575, y=w574) -> (x/y=w573:dbl)
        n161 = Divide(x=w573, y=8.854e-12) -> (x/y=w566:dbl)
        "K5k" <- w566
        "C5k" <- w570
        "tand5k" <- w565
      }
      frame #8 {
        n162 = flat-sequence {
          tunnel: w613 -> [w633]
          tunnel: [w632] -> _
          tunnel: [w631] -> w611
          tunnel: w612 -> [w630]
          tunnel: [w630] -> w615
          frame #0 {
            n163 = call-poly "VISA Configure Serial Port"("VISA resource name"=w633, "data bits (8)"=7, "parity (0:none)"=1) -> ("error out"=w638:errorcluster)  [unwired: 11 in, 1 out]
            n164 = Concatenate Strings("*X01", "\r") -> (w641:string)
            n165 = VISA Write(VISA resource name=w633, write buffer=w641, error in (no error)=w638) -> (VISA resource name out=w652:refnum<visa-resource-name>, error out=w642:errorcluster)  [unwired: 1 out]
            n166 = property class="Instr"(reference=w652, error in=w642) -> (error out=w643:errorcluster, "Serial Settings:Number of Bytes at Serial Port"=w644:u32)  [unwired: 1 out]
            n167 = VISA Read(VISA resource name=w633, byte count=w644, error in (no error)=w643) -> (read buffer=w645:string, error out=w632:errorcluster)  [unwired: 2 out]
            n168 = String Length(string=w645) -> (length=w647:i32)
            n169 = Subtract(x=w647, y=4) -> (x-y=w649:i32)
            n170 = String Subset(string=w645, offset (0)=3, length (rest)=w649) -> (substring=w650:string)
            n171 = Concatenate Strings(w650, "\t") -> (w634:string)
            n172 = Scan Value(string=w634, format string="%f") -> (value=w631:dbl)  [unwired: 1 in, 1 out]
            "Temp10kHz" <- w631
          }
        }
        n173 = flat-sequence {
          tunnel: w615 -> [w622]
          tunnel: [w624] -> w609
          tunnel: [w623] -> w614
          frame #0 {
            w621 = i16 0 items=["INTERNAL", "EXTERNAL", "HOLD/MANUAL"] ("trigger (internal:0)")
            w627 = i16 1 items=["DEG Q", "RAD D", "         R/G"] ("function B (deg q:0)")
            w628 = i16 3 items=["Z/Y", "R/G", "L", "C"] ("function A (z/y:0)")
            n174 = call "HP4192A Measure.vi"("OSC level (V)"=1.0, "test signal\nfreq (Hz)"="Freq Value (Hz) (10kHz)", "GPIB addess"=w622, "trigger (internal:0)"=w621, "function B (deg q:0)"=w627, "function A (z/y:0)"=w628) -> ("display B"=w624:dbl, "display A"=w623:dbl)  [unwired: 4 in]
            n175 = Wait (ms)(milliseconds to wait=u32 1000) -> ()  [unwired: 1 out]
          }
        }
        n176 = local read "Thickness"() -> (w620:dbl)
        n177 = local read "Area"() -> (w618:dbl)
        n178 = Multiply(x=w614, y=w620) -> (x*y=w619:dbl)
        n179 = Divide(x=w619, y=w618) -> (x/y=w617:dbl)
        n180 = Divide(x=w617, y=8.854e-12) -> (x/y=w610:dbl)
        "K10k" <- w610
        "C10k" <- w614
        "tand10k" <- w609
      }
      frame #9 {
        n181 = flat-sequence {
          tunnel: w657 -> [w677]
          tunnel: [w676] -> _
          tunnel: [w675] -> w655
          tunnel: w656 -> [w674]
          tunnel: [w674] -> w659
          frame #0 {
            n182 = call-poly "VISA Configure Serial Port"("VISA resource name"=w677, "data bits (8)"=7, "parity (0:none)"=1) -> ("error out"=w682:errorcluster)  [unwired: 11 in, 1 out]
            n183 = Concatenate Strings("*X01", "\r") -> (w685:string)
            n184 = VISA Write(VISA resource name=w677, write buffer=w685, error in (no error)=w682) -> (VISA resource name out=w696:refnum<visa-resource-name>, error out=w686:errorcluster)  [unwired: 1 out]
            n185 = property class="Instr"(reference=w696, error in=w686) -> (error out=w687:errorcluster, "Serial Settings:Number of Bytes at Serial Port"=w688:u32)  [unwired: 1 out]
            n186 = VISA Read(VISA resource name=w677, byte count=w688, error in (no error)=w687) -> (read buffer=w689:string, error out=w676:errorcluster)  [unwired: 2 out]
            n187 = String Length(string=w689) -> (length=w691:i32)
            n188 = Subtract(x=w691, y=4) -> (x-y=w693:i32)
            n189 = String Subset(string=w689, offset (0)=3, length (rest)=w693) -> (substring=w694:string)
            n190 = Concatenate Strings(w694, "\t") -> (w678:string)
            n191 = Scan Value(string=w678, format string="%f") -> (value=w675:dbl)  [unwired: 1 in, 1 out]
            "Temp25kHz" <- w675
          }
        }
        n192 = flat-sequence {
          tunnel: w659 -> [w666]
          tunnel: [w668] -> w653
          tunnel: [w667] -> w658
          frame #0 {
            w665 = i16 0 items=["INTERNAL", "EXTERNAL", "HOLD/MANUAL"] ("trigger (internal:0)")
            w671 = i16 1 items=["DEG Q", "RAD D", "         R/G"] ("function B (deg q:0)")
            w672 = i16 3 items=["Z/Y", "R/G", "L", "C"] ("function A (z/y:0)")
            n193 = call "HP4192A Measure.vi"("OSC level (V)"=1.0, "test signal\nfreq (Hz)"="Freq Value (Hz) (25kHz)", "GPIB addess"=w666, "trigger (internal:0)"=w665, "function B (deg q:0)"=w671, "function A (z/y:0)"=w672) -> ("display B"=w668:dbl, "display A"=w667:dbl)  [unwired: 4 in]
            n194 = Wait (ms)(milliseconds to wait=u32 1000) -> ()  [unwired: 1 out]
          }
        }
        n195 = local read "Thickness"() -> (w664:dbl)
        n196 = local read "Area"() -> (w662:dbl)
        n197 = Multiply(x=w658, y=w664) -> (x*y=w663:dbl)
        n198 = Divide(x=w663, y=w662) -> (x/y=w661:dbl)
        n199 = Divide(x=w661, y=8.854e-12) -> (x/y=w654:dbl)
        "K25k" <- w654
        "C25k" <- w658
        "tand25k" <- w653
      }
      frame #10 {
        n200 = flat-sequence {
          tunnel: w701 -> [w721]
          tunnel: [w720] -> _
          tunnel: [w719] -> w699
          tunnel: w700 -> [w718]
          tunnel: [w718] -> w703
          frame #0 {
            n201 = call-poly "VISA Configure Serial Port"("VISA resource name"=w721, "data bits (8)"=7, "parity (0:none)"=1) -> ("error out"=w726:errorcluster)  [unwired: 11 in, 1 out]
            n202 = Concatenate Strings("*X01", "\r") -> (w729:string)
            n203 = VISA Write(VISA resource name=w721, write buffer=w729, error in (no error)=w726) -> (VISA resource name out=w740:refnum<visa-resource-name>, error out=w730:errorcluster)  [unwired: 1 out]
            n204 = property class="Instr"(reference=w740, error in=w730) -> (error out=w731:errorcluster, "Serial Settings:Number of Bytes at Serial Port"=w732:u32)  [unwired: 1 out]
            n205 = VISA Read(VISA resource name=w721, byte count=w732, error in (no error)=w731) -> (read buffer=w733:string, error out=w720:errorcluster)  [unwired: 2 out]
            n206 = String Length(string=w733) -> (length=w735:i32)
            n207 = Subtract(x=w735, y=4) -> (x-y=w737:i32)
            n208 = String Subset(string=w733, offset (0)=3, length (rest)=w737) -> (substring=w738:string)
            n209 = Concatenate Strings(w738, "\t") -> (w722:string)
            n210 = Scan Value(string=w722, format string="%f") -> (value=w719:dbl)  [unwired: 1 in, 1 out]
            "Temp50kHz" <- w719
          }
        }
        n211 = flat-sequence {
          tunnel: w703 -> [w710]
          tunnel: [w713] -> w697
          tunnel: [w712] -> w702
          frame #0 {
            w709 = i16 0 items=["INTERNAL", "EXTERNAL", "HOLD/MANUAL"] ("trigger (internal:0)")
            w715 = i16 1 items=["DEG Q", "RAD D", "         R/G"] ("function B (deg q:0)")
            w716 = i16 3 items=["Z/Y", "R/G", "L", "C"] ("function A (z/y:0)")
            n212 = call "HP4192A Measure.vi"("OSC level (V)"=1.0, "test signal\nfreq (Hz)"="Freq Value (Hz) (50kHz)", "GPIB addess"=w710, "trigger (internal:0)"=w709, "function B (deg q:0)"=w715, "function A (z/y:0)"=w716) -> ("display B"=w713:dbl, "display A"=w712:dbl)  [unwired: 4 in]
            n213 = Wait (ms)(milliseconds to wait=u32 1000) -> ()  [unwired: 1 out]
          }
        }
        n214 = local read "Thickness"() -> (w708:dbl)
        n215 = local read "Area"() -> (w706:dbl)
        n216 = Multiply(x=w702, y=w708) -> (x*y=w707:dbl)
        n217 = Divide(x=w707, y=w706) -> (x/y=w705:dbl)
        n218 = Divide(x=w705, y=8.854e-12) -> (x/y=w698:dbl)
        "K50k" <- w698
        "C50k" <- w702
        "tand50k" <- w697
      }
      frame #11 {
        n219 = flat-sequence {
          tunnel: w745 -> [w765]
          tunnel: [w764] -> _
          tunnel: [w763] -> w743
          tunnel: w744 -> [w762]
          tunnel: [w762] -> w747
          frame #0 {
            n220 = call-poly "VISA Configure Serial Port"("VISA resource name"=w765, "data bits (8)"=7, "parity (0:none)"=1) -> ("error out"=w770:errorcluster)  [unwired: 11 in, 1 out]
            n221 = Concatenate Strings("*X01", "\r") -> (w773:string)
            n222 = VISA Write(VISA resource name=w765, write buffer=w773, error in (no error)=w770) -> (VISA resource name out=w784:refnum<visa-resource-name>, error out=w774:errorcluster)  [unwired: 1 out]
            n223 = property class="Instr"(reference=w784, error in=w774) -> (error out=w775:errorcluster, "Serial Settings:Number of Bytes at Serial Port"=w776:u32)  [unwired: 1 out]
            n224 = VISA Read(VISA resource name=w765, byte count=w776, error in (no error)=w775) -> (read buffer=w777:string, error out=w764:errorcluster)  [unwired: 2 out]
            n225 = String Length(string=w777) -> (length=w779:i32)
            n226 = Subtract(x=w779, y=4) -> (x-y=w781:i32)
            n227 = String Subset(string=w777, offset (0)=3, length (rest)=w781) -> (substring=w782:string)
            n228 = Concatenate Strings(w782, "\t") -> (w766:string)
            n229 = Scan Value(string=w766, format string="%f") -> (value=w763:dbl)  [unwired: 1 in, 1 out]
            "Temp100kHz" <- w763
          }
        }
        n230 = flat-sequence {
          tunnel: w747 -> [w754]
          tunnel: [w756] -> w741
          tunnel: [w755] -> w746
          frame #0 {
            w753 = i16 0 items=["INTERNAL", "EXTERNAL", "HOLD/MANUAL"] ("trigger (internal:0)")
            w759 = i16 1 items=["DEG Q", "RAD D", "         R/G"] ("function B (deg q:0)")
            w760 = i16 3 items=["Z/Y", "R/G", "L", "C"] ("function A (z/y:0)")
            n231 = call "HP4192A Measure.vi"("OSC level (V)"=1.0, "test signal\nfreq (Hz)"="Freq Value (Hz) (100kHz)", "GPIB addess"=w754, "trigger (internal:0)"=w753, "function B (deg q:0)"=w759, "function A (z/y:0)"=w760) -> ("display B"=w756:dbl, "display A"=w755:dbl)  [unwired: 4 in]
            n232 = Wait (ms)(milliseconds to wait=u32 1000) -> ()  [unwired: 1 out]
          }
        }
        n233 = local read "Thickness"() -> (w752:dbl)
        n234 = local read "Area"() -> (w750:dbl)
        n235 = Multiply(x=w746, y=w752) -> (x*y=w751:dbl)
        n236 = Divide(x=w751, y=w750) -> (x/y=w749:dbl)
        n237 = Divide(x=w749, y=8.854e-12) -> (x/y=w742:dbl)
        "K100k" <- w742
        "C100k" <- w746
        "tand100k" <- w741
      }
      frame #12 {
        n238 = flat-sequence {
          tunnel: w789 -> [w809]
          tunnel: [w808] -> _
          tunnel: [w807] -> w787
          tunnel: w788 -> [w806]
          tunnel: [w806] -> w791
          frame #0 {
            n239 = call-poly "VISA Configure Serial Port"("VISA resource name"=w809, "data bits (8)"=7, "parity (0:none)"=1) -> ("error out"=w814:errorcluster)  [unwired: 11 in, 1 out]
            n240 = Concatenate Strings("*X01", "\r") -> (w817:string)
            n241 = VISA Write(VISA resource name=w809, write buffer=w817, error in (no error)=w814) -> (VISA resource name out=w828:refnum<visa-resource-name>, error out=w818:errorcluster)  [unwired: 1 out]
            n242 = property class="Instr"(reference=w828, error in=w818) -> (error out=w819:errorcluster, "Serial Settings:Number of Bytes at Serial Port"=w820:u32)  [unwired: 1 out]
            n243 = VISA Read(VISA resource name=w809, byte count=w820, error in (no error)=w819) -> (read buffer=w821:string, error out=w808:errorcluster)  [unwired: 2 out]
            n244 = String Length(string=w821) -> (length=w823:i32)
            n245 = Subtract(x=w823, y=4) -> (x-y=w825:i32)
            n246 = String Subset(string=w821, offset (0)=3, length (rest)=w825) -> (substring=w826:string)
            n247 = Concatenate Strings(w826, "\t") -> (w810:string)
            n248 = Scan Value(string=w810, format string="%f") -> (value=w807:dbl)  [unwired: 1 in, 1 out]
            "Temp250kHz" <- w807
          }
        }
        n249 = flat-sequence {
          tunnel: w791 -> [w798]
          tunnel: [w801] -> w785
          tunnel: [w800] -> w790
          frame #0 {
            w797 = i16 0 items=["INTERNAL", "EXTERNAL", "HOLD/MANUAL"] ("trigger (internal:0)")
            w803 = i16 1 items=["DEG Q", "RAD D", "         R/G"] ("function B (deg q:0)")
            w804 = i16 3 items=["Z/Y", "R/G", "L", "C"] ("function A (z/y:0)")
            n250 = call "HP4192A Measure.vi"("OSC level (V)"=1.0, "test signal\nfreq (Hz)"="Freq Value (Hz) (250kHz)", "GPIB addess"=w798, "trigger (internal:0)"=w797, "function B (deg q:0)"=w803, "function A (z/y:0)"=w804) -> ("display B"=w801:dbl, "display A"=w800:dbl)  [unwired: 4 in]
            n251 = Wait (ms)(milliseconds to wait=u32 1000) -> ()  [unwired: 1 out]
          }
        }
        n252 = local read "Thickness"() -> (w796:dbl)
        n253 = local read "Area"() -> (w794:dbl)
        n254 = Multiply(x=w790, y=w796) -> (x*y=w795:dbl)
        n255 = Divide(x=w795, y=w794) -> (x/y=w793:dbl)
        n256 = Divide(x=w793, y=8.854e-12) -> (x/y=w786:dbl)
        "K250k" <- w786
        "C250k" <- w790
        "tand250k" <- w785
      }
      frame #13 {
        n257 = flat-sequence {
          tunnel: w833 -> [w853]
          tunnel: [w852] -> _
          tunnel: [w851] -> w831
          tunnel: w832 -> [w850]
          tunnel: [w850] -> w835
          frame #0 {
            n258 = call-poly "VISA Configure Serial Port"("VISA resource name"=w853, "data bits (8)"=7, "parity (0:none)"=1) -> ("error out"=w858:errorcluster)  [unwired: 11 in, 1 out]
            n259 = Concatenate Strings("*X01", "\r") -> (w861:string)
            n260 = VISA Write(VISA resource name=w853, write buffer=w861, error in (no error)=w858) -> (VISA resource name out=w872:refnum<visa-resource-name>, error out=w862:errorcluster)  [unwired: 1 out]
            n261 = property class="Instr"(reference=w872, error in=w862) -> (error out=w863:errorcluster, "Serial Settings:Number of Bytes at Serial Port"=w864:u32)  [unwired: 1 out]
            n262 = VISA Read(VISA resource name=w853, byte count=w864, error in (no error)=w863) -> (read buffer=w865:string, error out=w852:errorcluster)  [unwired: 2 out]
            n263 = String Length(string=w865) -> (length=w867:i32)
            n264 = Subtract(x=w867, y=4) -> (x-y=w869:i32)
            n265 = String Subset(string=w865, offset (0)=3, length (rest)=w869) -> (substring=w870:string)
            n266 = Concatenate Strings(w870, "\t") -> (w854:string)
            n267 = Scan Value(string=w854, format string="%f") -> (value=w851:dbl)  [unwired: 1 in, 1 out]
            "Temp500kHz" <- w851
          }
        }
        n268 = flat-sequence {
          tunnel: w835 -> [w842]
          tunnel: [w844] -> w829
          tunnel: [w843] -> w834
          frame #0 {
            w841 = i16 0 items=["INTERNAL", "EXTERNAL", "HOLD/MANUAL"] ("trigger (internal:0)")
            w847 = i16 1 items=["DEG Q", "RAD D", "         R/G"] ("function B (deg q:0)")
            w848 = i16 3 items=["Z/Y", "R/G", "L", "C"] ("function A (z/y:0)")
            n269 = call "HP4192A Measure.vi"("OSC level (V)"=1.0, "test signal\nfreq (Hz)"="Freq Value (Hz) (500kHz)", "GPIB addess"=w842, "trigger (internal:0)"=w841, "function B (deg q:0)"=w847, "function A (z/y:0)"=w848) -> ("display B"=w844:dbl, "display A"=w843:dbl)  [unwired: 4 in]
            n270 = Wait (ms)(milliseconds to wait=u32 1000) -> ()  [unwired: 1 out]
          }
        }
        n271 = local read "Thickness"() -> (w840:dbl)
        n272 = local read "Area"() -> (w838:dbl)
        n273 = Multiply(x=w834, y=w840) -> (x*y=w839:dbl)
        n274 = Divide(x=w839, y=w838) -> (x/y=w837:dbl)
        n275 = Divide(x=w837, y=8.854e-12) -> (x/y=w830:dbl)
        "K500k" <- w830
        "C500k" <- w834
        "tand500k" <- w829
      }
      frame #14 {
        n276 = flat-sequence {
          tunnel: w877 -> [w897]
          tunnel: [w896] -> _
          tunnel: [w895] -> w875
          tunnel: w876 -> [w894]
          tunnel: [w894] -> w879
          frame #0 {
            n277 = call-poly "VISA Configure Serial Port"("VISA resource name"=w897, "data bits (8)"=7, "parity (0:none)"=1) -> ("error out"=w902:errorcluster)  [unwired: 11 in, 1 out]
            n278 = Concatenate Strings("*X01", "\r") -> (w905:string)
            n279 = VISA Write(VISA resource name=w897, write buffer=w905, error in (no error)=w902) -> (VISA resource name out=w916:refnum<visa-resource-name>, error out=w906:errorcluster)  [unwired: 1 out]
            n280 = property class="Instr"(reference=w916, error in=w906) -> (error out=w907:errorcluster, "Serial Settings:Number of Bytes at Serial Port"=w908:u32)  [unwired: 1 out]
            n281 = VISA Read(VISA resource name=w897, byte count=w908, error in (no error)=w907) -> (read buffer=w909:string, error out=w896:errorcluster)  [unwired: 2 out]
            n282 = String Length(string=w909) -> (length=w911:i32)
            n283 = Subtract(x=w911, y=4) -> (x-y=w913:i32)
            n284 = String Subset(string=w909, offset (0)=3, length (rest)=w913) -> (substring=w914:string)
            n285 = Concatenate Strings(w914, "\t") -> (w898:string)
            n286 = Scan Value(string=w898, format string="%f") -> (value=w895:dbl)  [unwired: 1 in, 1 out]
            "Temp1MHz" <- w895
          }
        }
        n287 = flat-sequence {
          tunnel: w879 -> [w892]
          tunnel: [w886] -> w873
          tunnel: [w887] -> w878
          frame #0 {
            w885 = i16 0 items=["INTERNAL", "EXTERNAL", "HOLD/MANUAL"] ("trigger (internal:0)")
            w890 = i16 1 items=["DEG Q", "RAD D", "         R/G"] ("function B (deg q:0)")
            w891 = i16 3 items=["Z/Y", "R/G", "L", "C"] ("function A (z/y:0)")
            n288 = call "HP4192A Measure.vi"("OSC level (V)"=1.0, "test signal\nfreq (Hz)"="Freq Value (Hz) (1MHz)", "GPIB addess"=w892, "trigger (internal:0)"=w885, "function B (deg q:0)"=w890, "function A (z/y:0)"=w891) -> ("display B"=w886:dbl, "display A"=w887:dbl)  [unwired: 4 in]
            n289 = Wait (ms)(milliseconds to wait=u32 1000) -> ()  [unwired: 1 out]
          }
        }
        n290 = local read "Thickness"() -> (w884:dbl)
        n291 = local read "Area"() -> (w882:dbl)
        n292 = Multiply(x=w878, y=w884) -> (x*y=w883:dbl)
        n293 = Divide(x=w883, y=w882) -> (x/y=w881:dbl)
        n294 = Divide(x=w881, y=8.854e-12) -> (x/y=w874:dbl)
        "K1M" <- w874
        "C1M" <- w878
        "tand1M" <- w873
      }
    }
    n295 = flat-sequence {
      tunnel: w76 -> [w244]
      tunnel: w72 -> [w242]
      tunnel: w79 -> [w253]
      tunnel: w75 -> [w252]
      tunnel: w71 -> [w241]
      tunnel: w78 -> [w190]
      tunnel: w74 -> [w185]
      tunnel: w70 -> [w178]
      tunnel: w77 -> [w245]
      tunnel: w73 -> [w243]
      tunnel: w69 -> [w240]
      tunnel: w68 -> [w239]
      tunnel: w67 -> [w237]
      tunnel: w66 -> [w236]
      tunnel: w65 -> [w235]
      tunnel: w64 -> [w191]
      tunnel: w63 -> [w186]
      tunnel: w62 -> [w179]
      tunnel: w61 -> [w230]
      tunnel: w60 -> [w229]
      tunnel: w59 -> [w228]
      tunnel: w58 -> [w224]
      tunnel: w57 -> [w223]
      tunnel: w56 -> [w222]
      tunnel: w55 -> [w192]
      tunnel: w54 -> [w187]
      tunnel: w53 -> [w180]
      tunnel: w52 -> [w218]
      tunnel: w51 -> [w217]
      tunnel: w50 -> [w216]
      tunnel: w49 -> [w213]
      tunnel: w48 -> [w212]
      tunnel: w47 -> [w211]
      tunnel: w46 -> [w193]
      tunnel: w45 -> [w188]
      tunnel: w44 -> [w181]
      tunnel: w43 -> [w206]
      tunnel: w42 -> [w205]
      tunnel: w41 -> [w204]
      tunnel: w40 -> [w184]
      tunnel: w39 -> [w183]
      tunnel: w38 -> [w182]
      tunnel: w37 -> [w199]
      tunnel: w36 -> [w189]
      tunnel: w35 -> [w194]
      tunnel: [w184] -> w34
      tunnel: [w193] -> w33
      tunnel: [w192] -> w32
      tunnel: [w191] -> w31
      tunnel: [w190] -> w30
      tunnel: [w183] -> w29
      tunnel: [w188] -> w28
      tunnel: [w187] -> w27
      tunnel: [w186] -> w26
      tunnel: [w185] -> w25
      tunnel: [w182] -> w24
      tunnel: [w181] -> w23
      tunnel: [w180] -> w22
      tunnel: [w179] -> w21
      tunnel: [w178] -> w20
      frame #0 {
        w197 = 1000000000000.0 ("x")
        n296 = local read "C2.5k"() -> (w226:dbl)
        n297 = local read "C100k"() -> (w207:dbl)
        n298 = local read "C250k"() -> (w202:dbl)
        n299 = local read "C500k"() -> (w200:dbl)
        n300 = local read "C250"() -> (w233:dbl)
        n301 = local read "C10k"() -> (w219:dbl)
        n302 = local read "C25"() -> (w251:dbl)
        n303 = local read "C500"() -> (w238:dbl)
        n304 = local read "C25k"() -> (w214:dbl)
        n305 = local read "C100"() -> (w234:dbl)
        n306 = local read "C50k"() -> (w209:dbl)
        n307 = local read "C50"() -> (w246:dbl)
        n308 = local read "C1k"() -> (w231:dbl)
        n309 = local read "C5k"() -> (w221:dbl)
        n310 = local read "C1M"() -> (w196:dbl)
        n311 = Multiply(x=w197, y=w251) -> (x*y=w250:dbl)
        n312 = Multiply(x=w197, y=w246) -> (x*y=w249:dbl)
        n313 = Multiply(x=w197, y=w234) -> (x*y=w248:dbl)
        n314 = Multiply(x=w197, y=w238) -> (x*y=w232:dbl)
        n315 = Multiply(x=w197, y=w233) -> (x*y=w247:dbl)
        n316 = Multiply(x=w197, y=w231) -> (x*y=w227:dbl)
        n317 = Multiply(x=w197, y=w226) -> (x*y=w225:dbl)
        n318 = Multiply(x=w197, y=w221) -> (x*y=w220:dbl)
        n319 = Multiply(x=w197, y=w219) -> (x*y=w215:dbl)
        n320 = Multiply(x=w197, y=w214) -> (x*y=w210:dbl)
        n321 = Multiply(x=w197, y=w209) -> (x*y=w208:dbl)
        n322 = Multiply(x=w197, y=w207) -> (x*y=w203:dbl)
        n323 = Multiply(x=w197, y=w202) -> (x*y=w201:dbl)
        n324 = Multiply(x=w197, y=w200) -> (x*y=w198:dbl)
        n325 = Multiply(x=w197, y=w196) -> (x*y=w195:dbl)
        n326 = Build Array(w239, w250, w244, w242, w253, w249, w252, w241, w190, w248, w185, w178, w245, w247, w243, w240, w237, w232, w236, w235, w191, w227, w186, w179, w230, w225, w229, w228, w224, w220, w223, w222, w192, w215, w187, w180, w218, w210, w217, w216, w213, w208, w212, w211, w193, w203, w188, w181, w206, w201, w205, w204, w184, w198, w183, w182, w194, w195, w189, w199) -> (w256:dbl[])
        n327 = local read "Path & File Name (*.txt)"() -> (w254:path)
        n328 = call-poly <vilib>:"Write To Spreadsheet File.vi"("format (%.3f)"="%.10f", "append to file? (new file:F)"=TRUE, "1D data"=w256, "file path (dialog if empty)"=w254) -> ()  [unwired: 4 in, 1 out]
      }
    }
    n329 = flat-sequence {
      tunnel: w30 -> [w143]
      tunnel: w31 -> [w142]
      tunnel: w32 -> [w141]
      tunnel: w33 -> [w140]
      tunnel: w25 -> [w139]
      tunnel: w26 -> [w138]
      tunnel: w27 -> [w137]
      tunnel: w28 -> [w136]
      tunnel: w20 -> [w135]
      tunnel: w21 -> [w134]
      tunnel: w22 -> [w133]
      tunnel: w23 -> [w132]
      tunnel: w34 -> [w96]
      tunnel: w29 -> [w88]
      tunnel: w24 -> [w81]
      frame #0 {
        n330 = Insert Into Array(array="Temp10k", index=0, new element=w141) -> (w103:dbl[])
        n331 = Insert Into Array(array="Temp500k", index=0, new element=w96) -> (w93:dbl[])
        n332 = Insert Into Array(array="Temp100", index=0, new element=w143) -> (w105:dbl[])
        n333 = Insert Into Array(array="Temp1k", index=0, new element=w142) -> (w104:dbl[])
        n334 = Insert Into Array(array="Temp100k", index=0, new element=w140) -> (w102:dbl[])
        n335 = Insert Into Array(array="K100", index=0, new element=w139) -> (w125:dbl[])
        n336 = Insert Into Array(array="K10k", index=0, new element=w137) -> (w123:dbl[])
        n337 = Insert Into Array(array="K500k", index=0, new element=w88) -> (w87:dbl[])
        n338 = Insert Into Array(array="K1k", index=0, new element=w138) -> (w124:dbl[])
        n339 = Insert Into Array(array="K100k", index=0, new element=w136) -> (w122:dbl[])
        n340 = Build Array(w104) -> (w119:dbl[][])
        n341 = Build Array(w103) -> (w117:dbl[][])
        n342 = Build Array(w102) -> (w115:dbl[][])
        n343 = Build Array(w93) -> (w98:dbl[][])
        n344 = Build Array(w105) -> (w121:dbl[][])
        n345 = call "Convert to Dynamic Data19"("Array"=w87) -> ("Dynamic Data Type"=w91:dynamicdata)  [unwired: 3 in]
        n346 = Build Array(w104) -> (w108:dbl[][])
        n347 = Build Array(w103) -> (w110:dbl[][])
        n348 = Build Array(w102) -> (w112:dbl[][])
        n349 = Build Array(w93) -> (w92:dbl[][])
        n350 = call "Convert to Dynamic Data5"("Array"=w125) -> ("Dynamic Data Type"=w131:dynamicdata)  [unwired: 3 in]
        n351 = call "Convert to Dynamic Data6"("Array"=w124) -> ("Dynamic Data Type"=w130:dynamicdata)  [unwired: 3 in]
        n352 = call "Convert to Dynamic Data7"("Array"=w123) -> ("Dynamic Data Type"=w129:dynamicdata)  [unwired: 3 in]
        n353 = call "Convert to Dynamic Data8"("Array"=w122) -> ("Dynamic Data Type"=w128:dynamicdata)  [unwired: 3 in]
        n354 = Build Array(w105) -> (w106:dbl[][])
        n355 = Insert Into Array(array="tand100", index=0, new element=w135) -> (w161:dbl[])
        n356 = Insert Into Array(array="tand1k", index=0, new element=w134) -> (w162:dbl[])
        n357 = Insert Into Array(array="tand10k", index=0, new element=w133) -> (w163:dbl[])
        n358 = Insert Into Array(array="tand100k", index=0, new element=w132) -> (w164:dbl[])
        n359 = Insert Into Array(array="tand500k", index=0, new element=w81) -> (w82:dbl[])
        n360 = call "Convert to Dynamic Data9"("Array"=w161) -> ("Dynamic Data Type"=w146:dynamicdata)  [unwired: 3 in]
        n361 = call "Convert to Dynamic Data10"("Array"=w162) -> ("Dynamic Data Type"=w147:dynamicdata)  [unwired: 3 in]
        n362 = call "Convert to Dynamic Data11"("Array"=w163) -> ("Dynamic Data Type"=w100:dynamicdata)  [unwired: 3 in]
        n363 = call "Convert to Dynamic Data12"("Array"=w164) -> ("Dynamic Data Type"=w86:dynamicdata)  [unwired: 3 in]
        n364 = call "Convert to Dynamic Data20"("Array"=w82) -> ("Dynamic Data Type"=w85:dynamicdata)  [unwired: 3 in]
        n365 = call "Convert to Dynamic Data13"("2D Array"=w121) -> ("Dynamic Data Type"=w120:dynamicdata)  [unwired: 3 in]
        n366 = call "Convert to Dynamic Data"("2D Array"=w119) -> ("Dynamic Data Type"=w118:dynamicdata)  [unwired: 3 in]
        n367 = call "Convert to Dynamic Data2"("2D Array"=w117) -> ("Dynamic Data Type"=w116:dynamicdata)  [unwired: 3 in]
        n368 = call "Convert to Dynamic Data3"("2D Array"=w115) -> ("Dynamic Data Type"=w114:dynamicdata)  [unwired: 3 in]
        n369 = call "Convert to Dynamic Data17"("2D Array"=w98) -> ("Dynamic Data Type"=w99:dynamicdata)  [unwired: 3 in]
        n370 = call "Convert to Dynamic Data4"("2D Array"=w106) -> ("Dynamic Data Type"=w107:dynamicdata)  [unwired: 3 in]
        n371 = call "Convert to Dynamic Data14"("2D Array"=w108) -> ("Dynamic Data Type"=w109:dynamicdata)  [unwired: 3 in]
        n372 = call "Convert to Dynamic Data15"("2D Array"=w110) -> ("Dynamic Data Type"=w111:dynamicdata)  [unwired: 3 in]
        n373 = call "Convert to Dynamic Data16"("2D Array"=w112) -> ("Dynamic Data Type"=w113:dynamicdata)  [unwired: 3 in]
        n374 = call "Convert to Dynamic Data18"("2D Array"=w92) -> ("Dynamic Data Type"=w94:dynamicdata)  [unwired: 3 in]
        n375 = Merge Signals(w120, w118, w116, w114, w99) -> (w126:dynamicdata)
        n376 = Merge Signals(w131, w130, w129, w128, w91) -> (w127:dynamicdata)
        n377 = Merge Signals(w107, w109, w111, w113, w94) -> (w101:dynamicdata)
        n378 = Merge Signals(w146, w147, w100, w86, w85) -> (w148:dynamicdata)
        n379 = call "Build XY Graph"("Y Input"=w127, "X Input"=w126) -> ("XY Graph"=→"Relative Permittivity vs. Temperature":cluster{"Y":dbl[], "Y":dbl[]}[])  [unwired: 8 in, 1 out]
        n380 = call "Build XY Graph2"("Y Input"=w148, "X Input"=w101) -> ("XY Graph"=→"Dielectric Loss vs. Temperature":cluster{"Y":dbl[], "Y":dbl[]}[])  [unwired: 8 in, 1 out]
      }
    }
  }
  n381 = flat-sequence {
    tunnel: w2 -> [w978]
    tunnel: [w976] -> w1
    frame #0 {
      w945 = "\t"
      w946 = "Temperature (C)" ("string")
      n382 = local read "Thickness"() -> (w982:dbl)
      n383 = local read "Area"() -> (w983:dbl)
      n384 = Number To Exponential String(number=w983) -> (E-format string=w975:string)  [unwired: 3 in]
      n385 = Number To Exponential String(number=w982) -> (E-format string=w973:string)  [unwired: 3 in]
      n386 = Concatenate Strings("Thickness (m)" ("string"), "\t", w973) -> (w971:string)
      n387 = Concatenate Strings("Area (m^2)" ("string"), "\t", w975) -> (w979:string)
      n388 = Concatenate Strings("Comment" ("string"), "\t", "Comment (Sample's Name, compositions, whatever you want,..)", "\r", w979, "\t", w971, "\r", w946, w945, "C25Hz (pF)" ("string"), w945, "K25Hz" ("string"), w945, "tand25Hz" ("string"), w945, w946, w945, "C50Hz (pF)" ("string"), w945, "K50Hz" ("string"), w945, "tand50Hz" ("string"), w945, w946, w945, "C100Hz (pF)" ("string"), w945, "K100Hz" ("string"), w945, "tand100Hz" ("string"), w945, w946, w945, "C250Hz (pF)" ("string"), w945, "K250Hz" ("string"), w945, "tand250Hz" ("string"), w945, w946, w945, "C500Hz (pF)" ("string"), w945, "K500Hz" ("string"), w945, "tand500Hz" ("string"), w945, w946, w945, "C1kHz (pF)" ("string"), w945, "K1kHz" ("string"), w945, "tand1kHz" ("string"), w945, w946, w945, "C2.5kHz (pF)" ("string"), w945, "K2.5kHz" ("string"), w945, "tand2.5kHz" ("string"), w945, w946, w945, "C5kHz (pF)" ("string"), w945, "K5kHz" ("string"), w945, "tand5kHz" ("string"), w945, w946, w945, "C10kHz (pF)" ("string"), w945, "K10kHz" ("string"), w945, "tand10kHz" ("string"), w945, w946, w945, "C25kHz (pF)" ("string"), w945, "K25kHz" ("string"), w945, "tand25kHz" ("string"), w945, w946, w945, "C50kHz (pF)" ("string"), w945, "K50kHz" ("string"), w945, "tand50kHz" ("string"), w945, w946, w945, "C100kHz (pF)" ("string"), w945, "K100kHz" ("string"), w945, "tand100kHz" ("string"), w945, w946, w945, "C250kHz (pF)" ("string"), w945, "K250kHz" ("string"), w945, "tand250kHz" ("string"), w945, w946, w945, "C500kHz (pF)" ("string"), w945, "K500kHz" ("string"), w945, "tand500kHz" ("string"), w945, w946, w945, "C1MHz (pF)" ("string"), w945, "K1MHz" ("string"), w945, "tand1MHz" ("string"), "\r\n") -> (w977:string)
      n389 = Write to Text File(file (use dialog)=w978, text=w977) -> (error out=w976:errorcluster)  [unwired: 2 in, 2 out]
    }
  }
